vi "Autonomous Independent.vi"   [LabVIEW 2015]
doc: "This VI is called when autonomous begins, and will automatically be terminated when autonomous ends. You can carry out timed or sensor driven robot movement independently without needing to return to the caller."
uses:
  <vilib>/Rock Robotics/WPI/CAN/TalonSRX/WPI_CANTalonSRX_APIFeedbackSelect.ctl
  <vilib>/Rock Robotics/WPI/CAN/TalonSRX/WPI_CANTalonSRX_APIControlMode.ctl
  <vilib>/Rock Robotics/Network Tables/SD Read Number.vi
  <vilib>/Rock Robotics/WPI/Utilities/WPI_GetSetVariantRefNum.vi
  <vilib>/Rock Robotics/Network Tables/NT Read Number.vi
  <vilib>/Rock Robotics/WPI/RobotDrive/WPI_RobotDriveArcadeDrive_Standard(NoSaturation).vi
panel:
  # "Be sure to right-click and choose Data Operations>>Make Current Value default if you want to save the array values with the VI"
types:
  T1 = typedef "WPI_MotorControlDeviceRef.ctl" = cluster{"DeviceStatus":errorcluster, "Type":T2, "PWM":cluster{"PWM Channel":T3, "DeadBand":T4}, "CAN":cluster{"Device Number":u8, "Control Mode":T5, "Semaphore":T6, "Max Vout":dbl, "TalonSRX Control Mode":T7}, "Invert":bool}
  T2 = typedef "WPI_MotorControlType.ctl" = enum16{"PWM", "CAN", "CANTalonSRX"}
  T3 = typedef "FPGA_DIOPWMChannel.ctl" = enum8{"PWM 0", "PWM 1", "PWM 2", "PWM 3", "PWM 4", "PWM 5", "PWM 6", "PWM 7", "PWM 8", "PWM 9", "PWM MXP 0", "PWM MXP 1", "PWM MXP 2", "PWM MXP 3", "PWM MXP 4", "PWM MXP 5", "PWM MXP 6", "PWM MXP 7", "PWM MXP 8", "PWM MXP 9", "Invalid"}
  T4 = typedef "WPI_PWMDeadband.ctl" = cluster{"Name":string, "maxPositivePwm":i32, "minPositivePwm":i32, "centerPwm":i32, "maxNegativePwm":i32, "minNegativePwm":i32, "angularRange":u16}
  T5 = typedef "WPI_CANJaguar_ControlMode.ctl" = enum8{"Percent VBus", "Current", "Speed", "Position", "Voltage"}
  T6 = typedef "Semaphore RefNum" = refnum<k1>
  T7 = typedef "WPI_CANTalonSRX_APIControlMode.ctl" = enum8{"Percent VBus", "Speed", "Position", "Slave", "Unchanged / Invalid", "Voltage Compensation", "Current", "Motion Profile"}
  T8 = typedef "WPI_SwitchDevRef.ctl" = cluster{"DevStatus":errorcluster, "DIO Channel":T9, "CntIndex":T10, "Normally Closed":bool}
  T9 = typedef "FPGA_DIOChannel.ctl" = enum8{"DIO 0", "DIO 1", "DIO 2", "DIO 3", "DIO 4", "DIO 5", "DIO 6", "DIO 7", "DIO 8", "DIO 9", "DIO MXP 0", "DIO MXP 1", "DIO MXP 2", "DIO MXP 3", "DIO MXP 4", "DIO MXP 5", "DIO MXP 6", "DIO MXP 7", "DIO MXP 8", "DIO MXP 9", "DIO MXP 10", "DIO MXP 11", "DIO MXP 12", "DIO MXP 13", "DIO MXP 14", "DIO MXP 15", "Invalid"}
  T10 = typedef "FPGA_CounterCtrSystemIndex.ctl" = enum8{"Ctr 0", "Ctr 1", "Ctr 2", "Ctr 3", "Ctr 4", "Ctr 5", "Ctr 6", "Ctr 7", "Invalid"}
  T11 = typedef "WPI_GyroDevRef.ctl" = cluster{"DevStatus":errorcluster, "Analog Channel":T12, "Offset":dbl, "Gain (VoltsPerDegree/Second)":dbl, "Gyro Type":enum16{"Analog", "XRS450"}, "Handle":i32, "SPI Bus":T13, "Device Found":bool, "Sample Rate":dbl, "Calibrate On Open":bool}
  T12 = typedef "FPGA_AIChannel.ctl" = enum8{"AI 0", "AI 1", "AI 2", "AI 3", "AI MXP 0", "AI MXP 1", "AI MXP 2", "AI MXP 3", "Invalid"}
  T13 = typedef "spi_bus.ctl" = enum16{"SPI On-Board, CS0", "SPI On-Board, CS1", "SPI On-Board, CS2", "SPI On-Board, CS3", "SPI MXP", "Invalid"}
  T14 = typedef "WPI_RobotDriveDevRef.ctl" = cluster{"DevStatus":errorcluster, "Motors[]":T1[], "Square Inputs":bool, "Max Output":dbl}
  T15 = typedef "WPI_EncoderDevRef.ctl" = cluster{"DevStatus":errorcluster, "EncoderIndex":T16, "CounterIndex":T10, "DistancePerCount":dbl, "Decoding Type":T17}
  T16 = typedef "FPGA_EncoderIdx.ctl" = enum8{"Enc 0", "Enc 1", "Enc 2", "Enc 3", "Enc 4", "Enc 5", "Enc 6", "Enc 7", "Invalid"}
  T17 = typedef "WPI_EncoderType.ctl" = enum16{"1x", "2x", "4x"}
  T18 = typedef "WPI_CANTalonSRX_APIFeedbackSelect.ctl" = enum16{"Digital Quadrature Encoder", "Analog Potentiometer", "Analog Encoder", "Count on Quad-A (Rising-Edge)", "Count on Quad-A (Falling-Edge)", "CTR Magnetic Enc (Absolute)", "CTR Magnetic Enc (Relative)", "Pulse Width"}
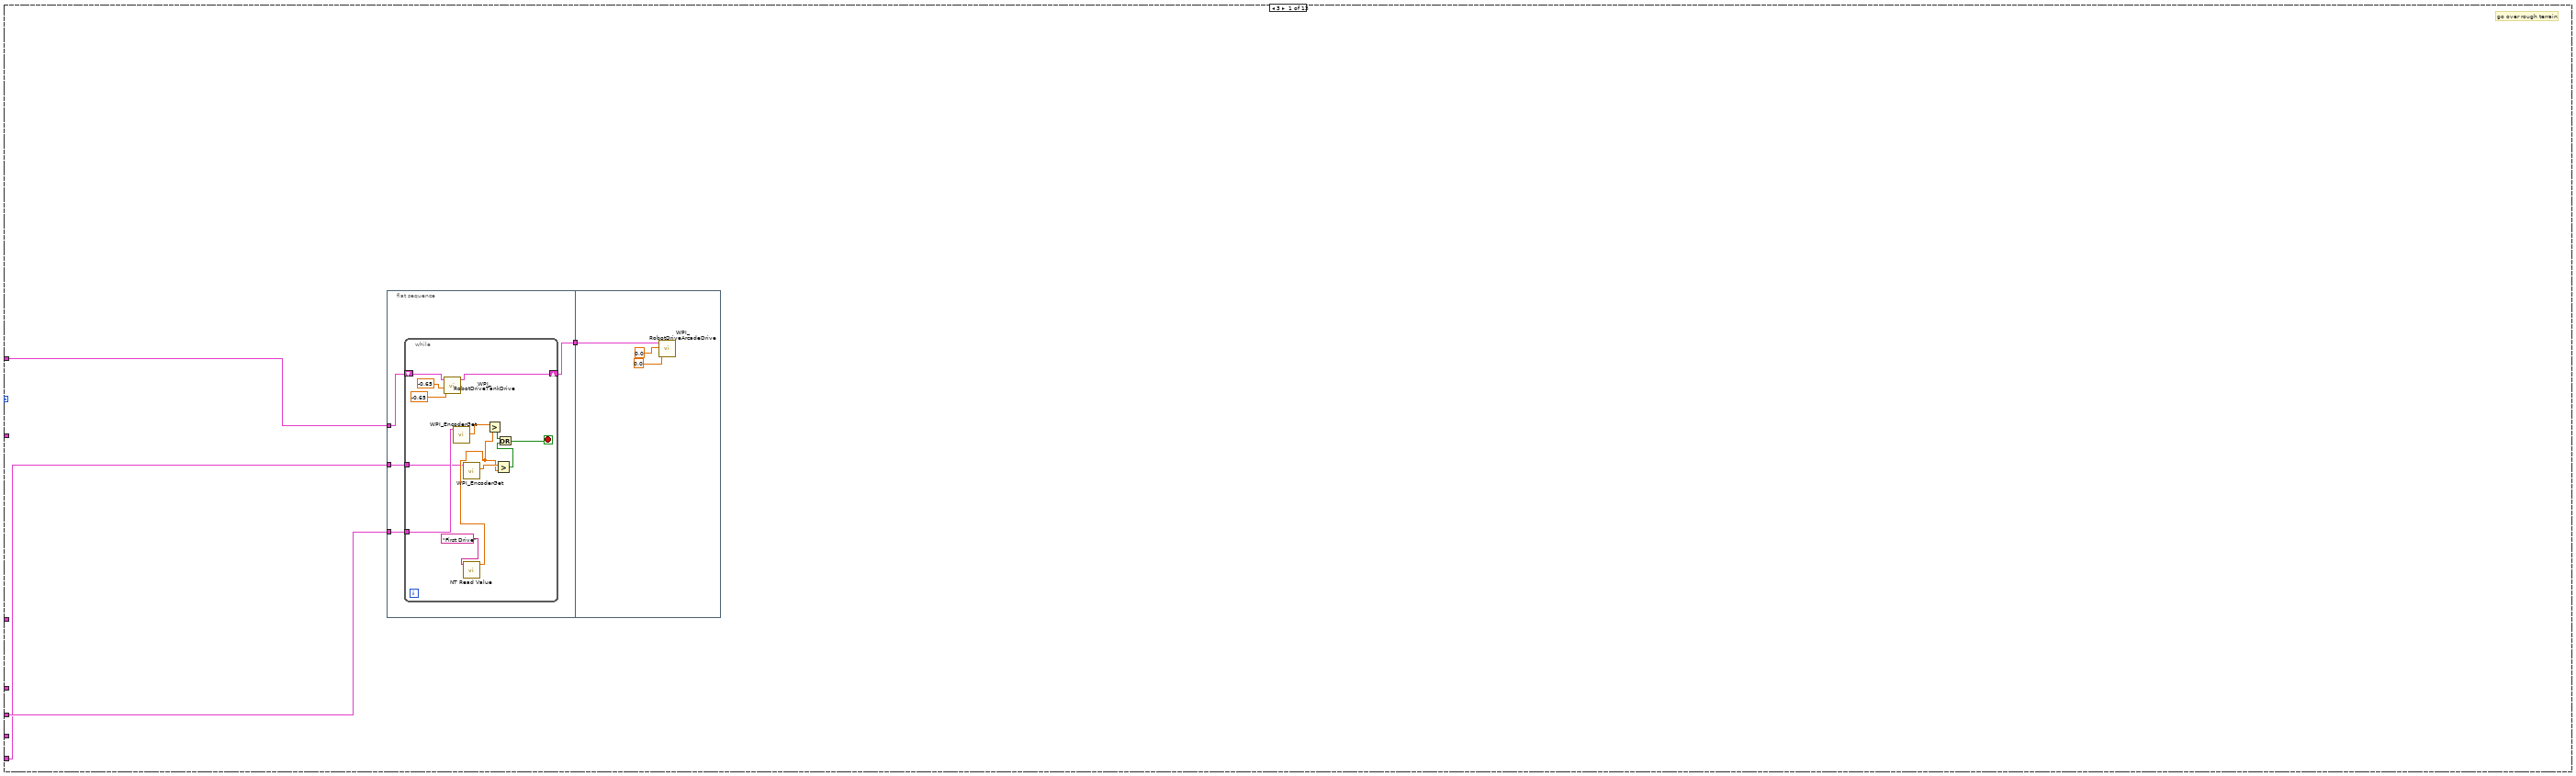
[diagram p2: hidden frame]
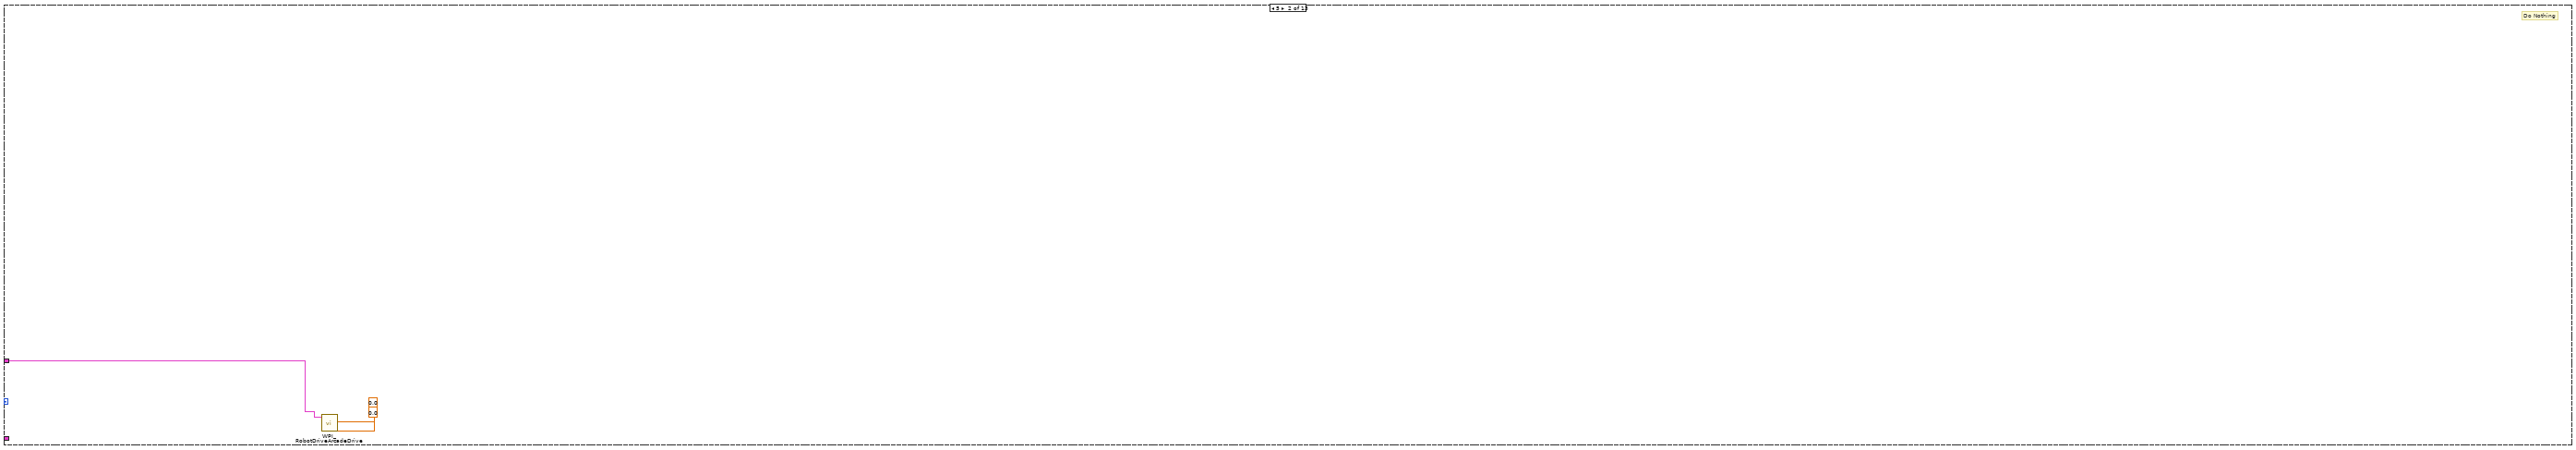
[diagram p3: hidden frame]
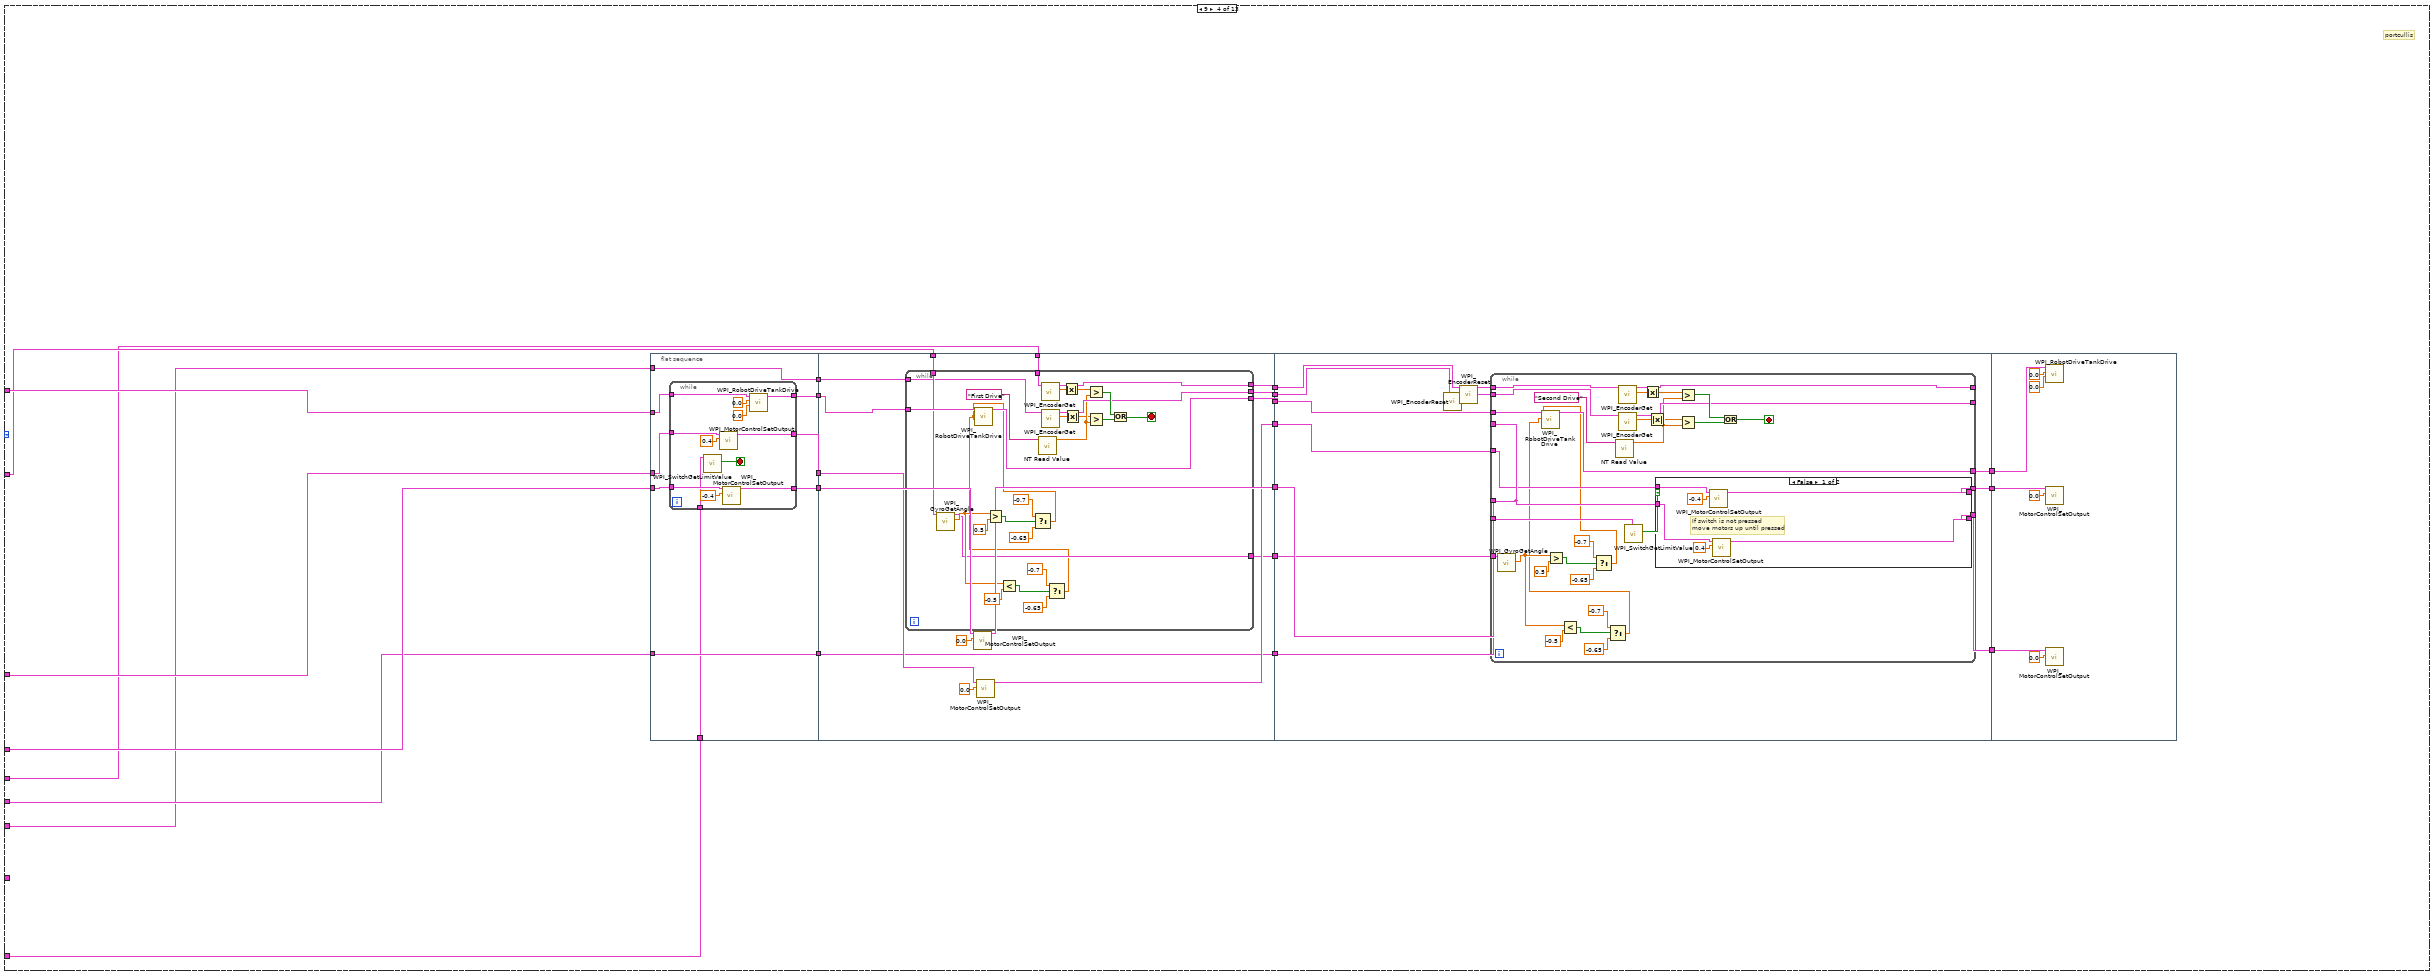
[diagram p4: hidden frame]
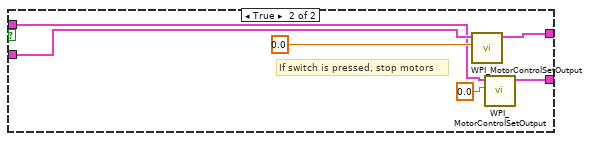
[diagram p5: hidden frame]
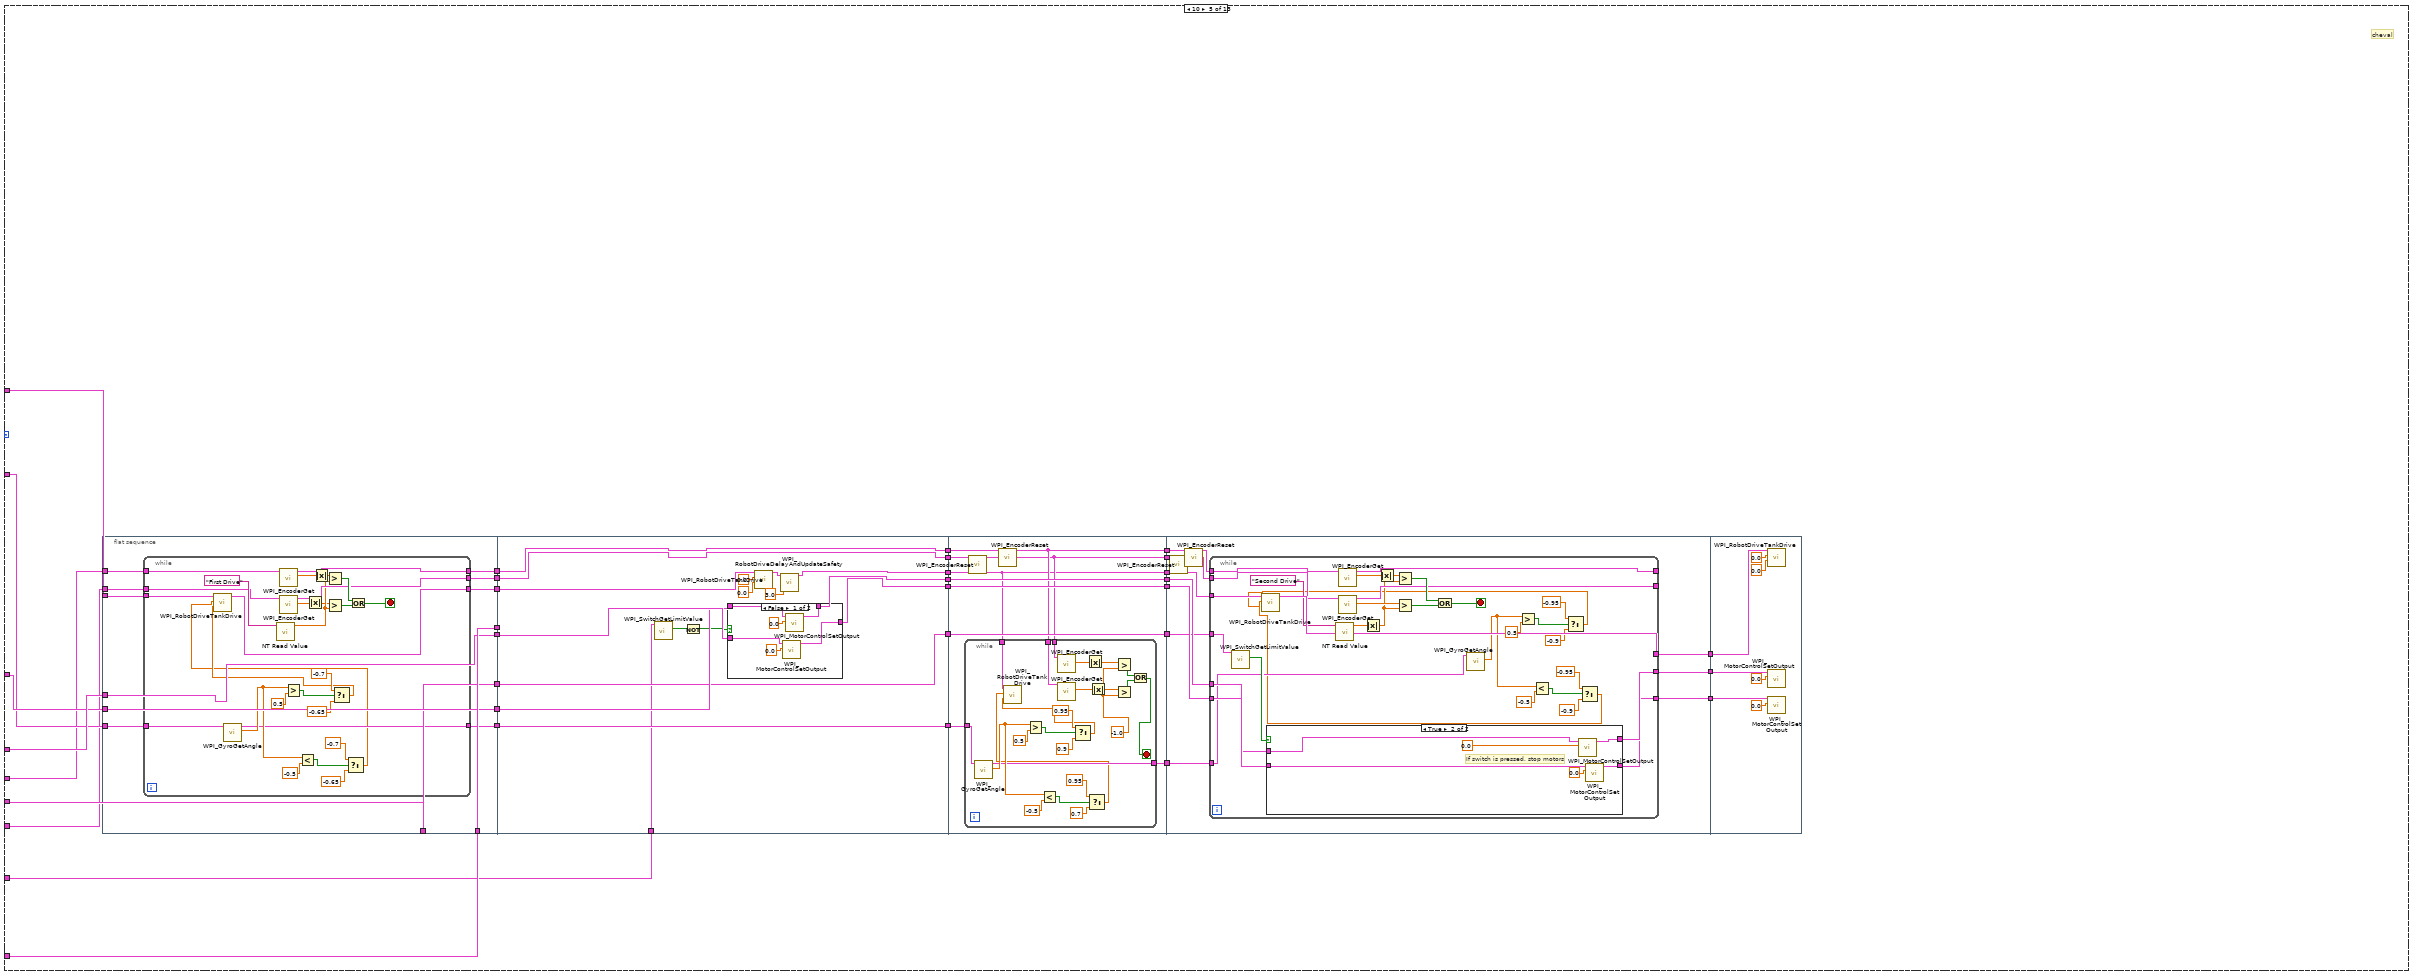
[diagram p6: hidden frame]
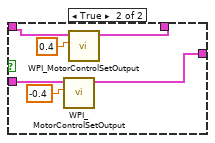
[diagram p7: hidden frame]
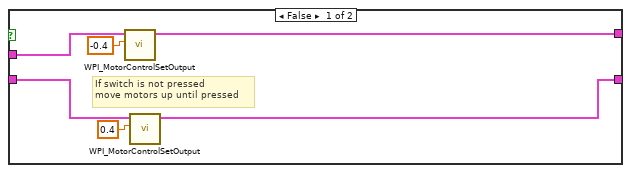
[diagram p8: hidden frame]
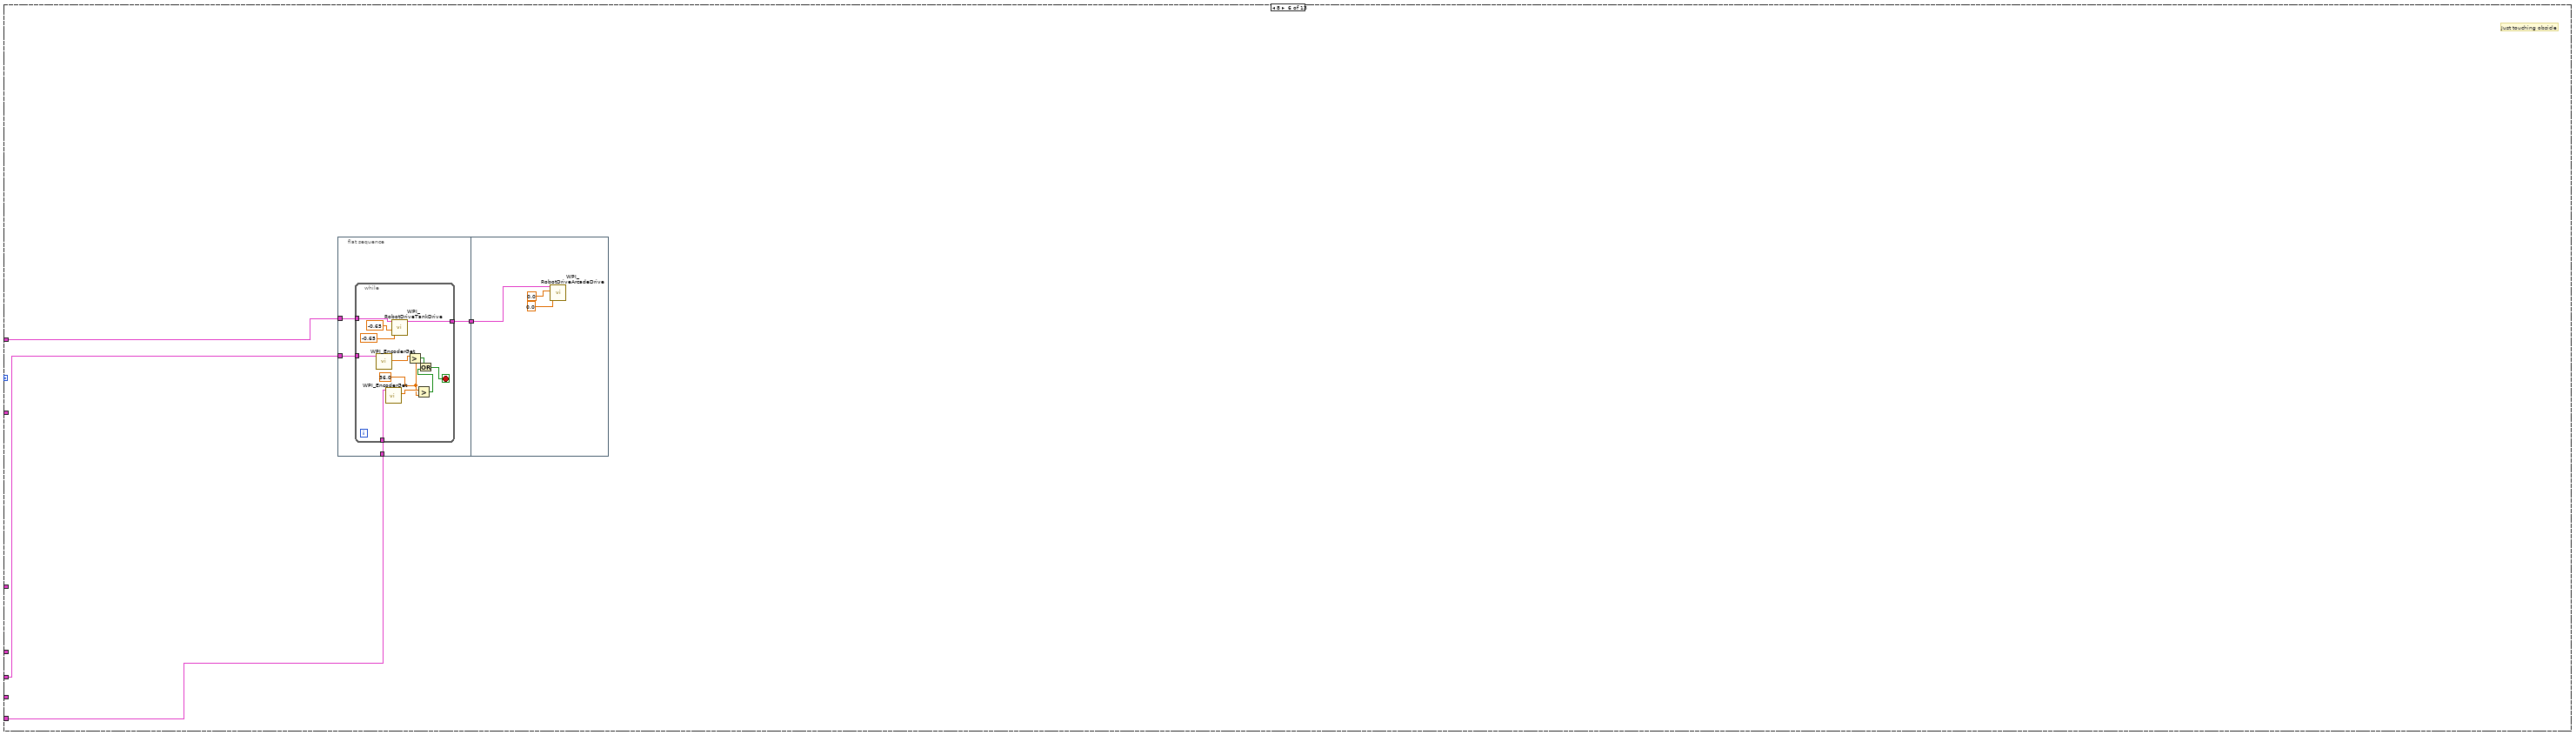
[diagram p9: hidden frame]
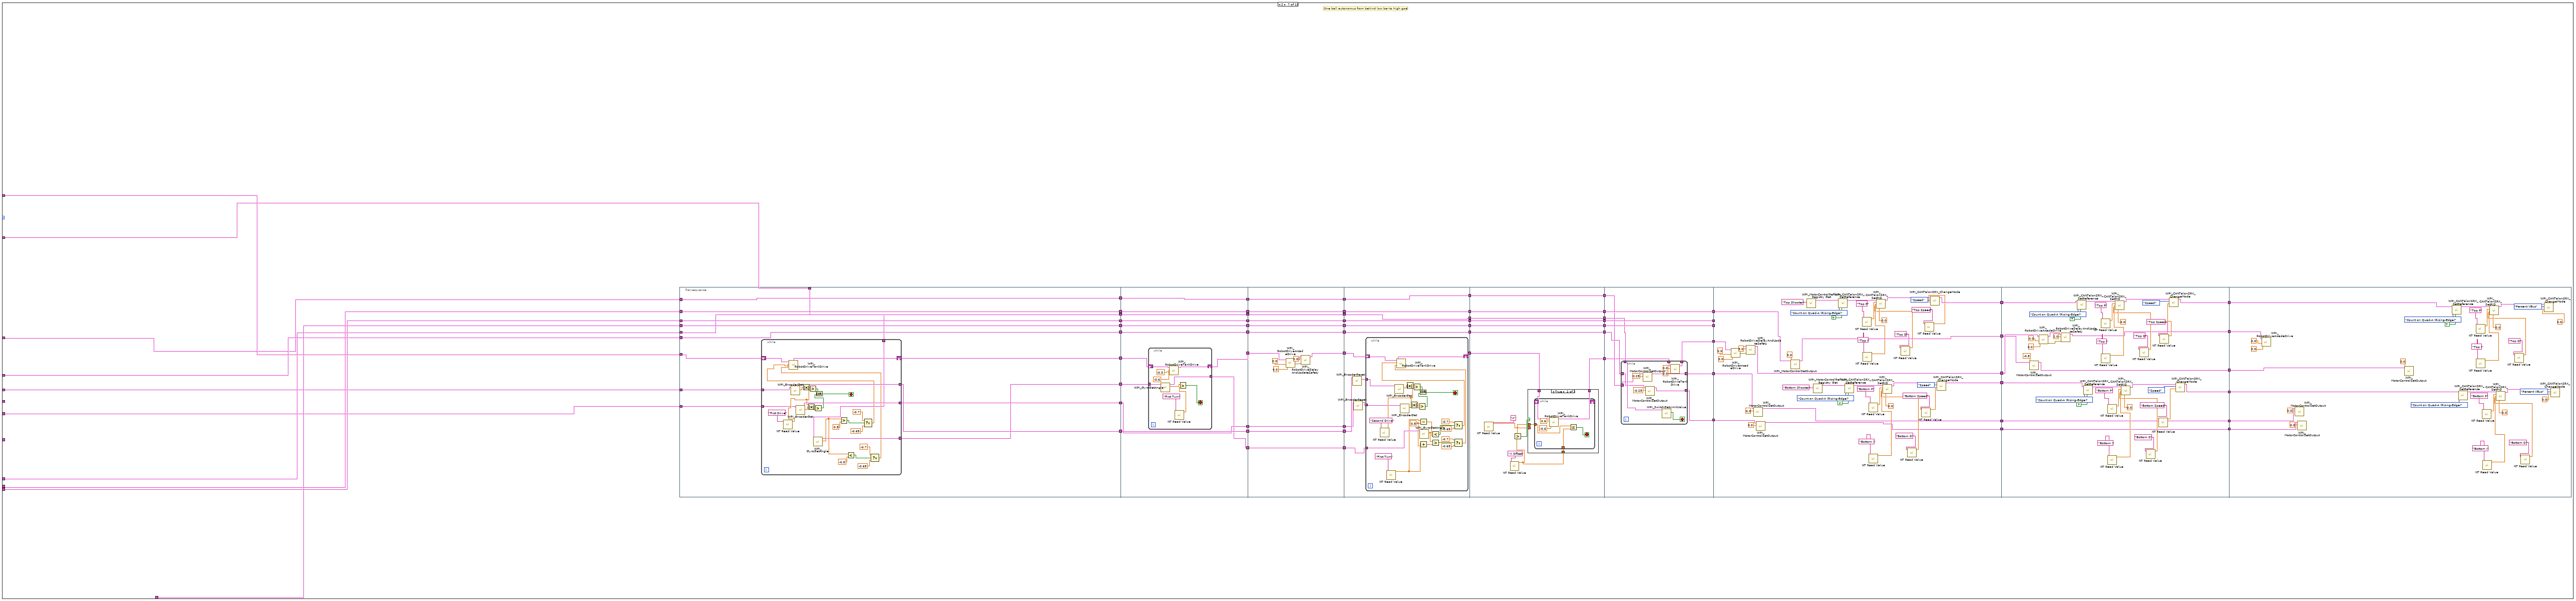
[diagram p10: hidden frame]
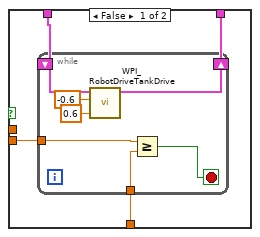
[diagram p11: hidden frame]
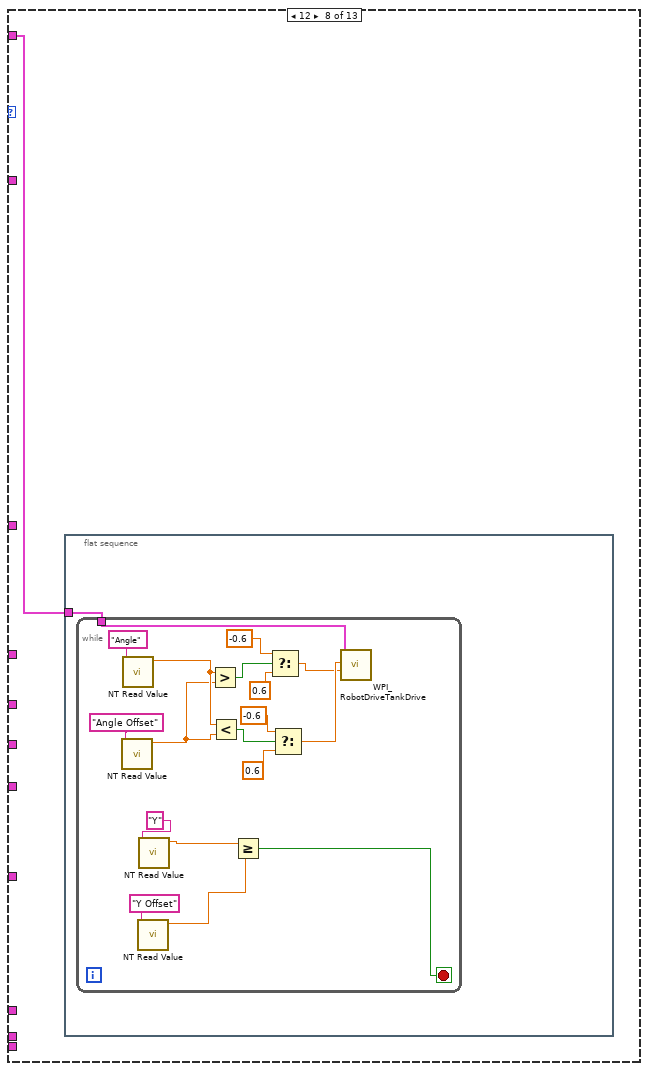
[diagram p12: hidden frame]
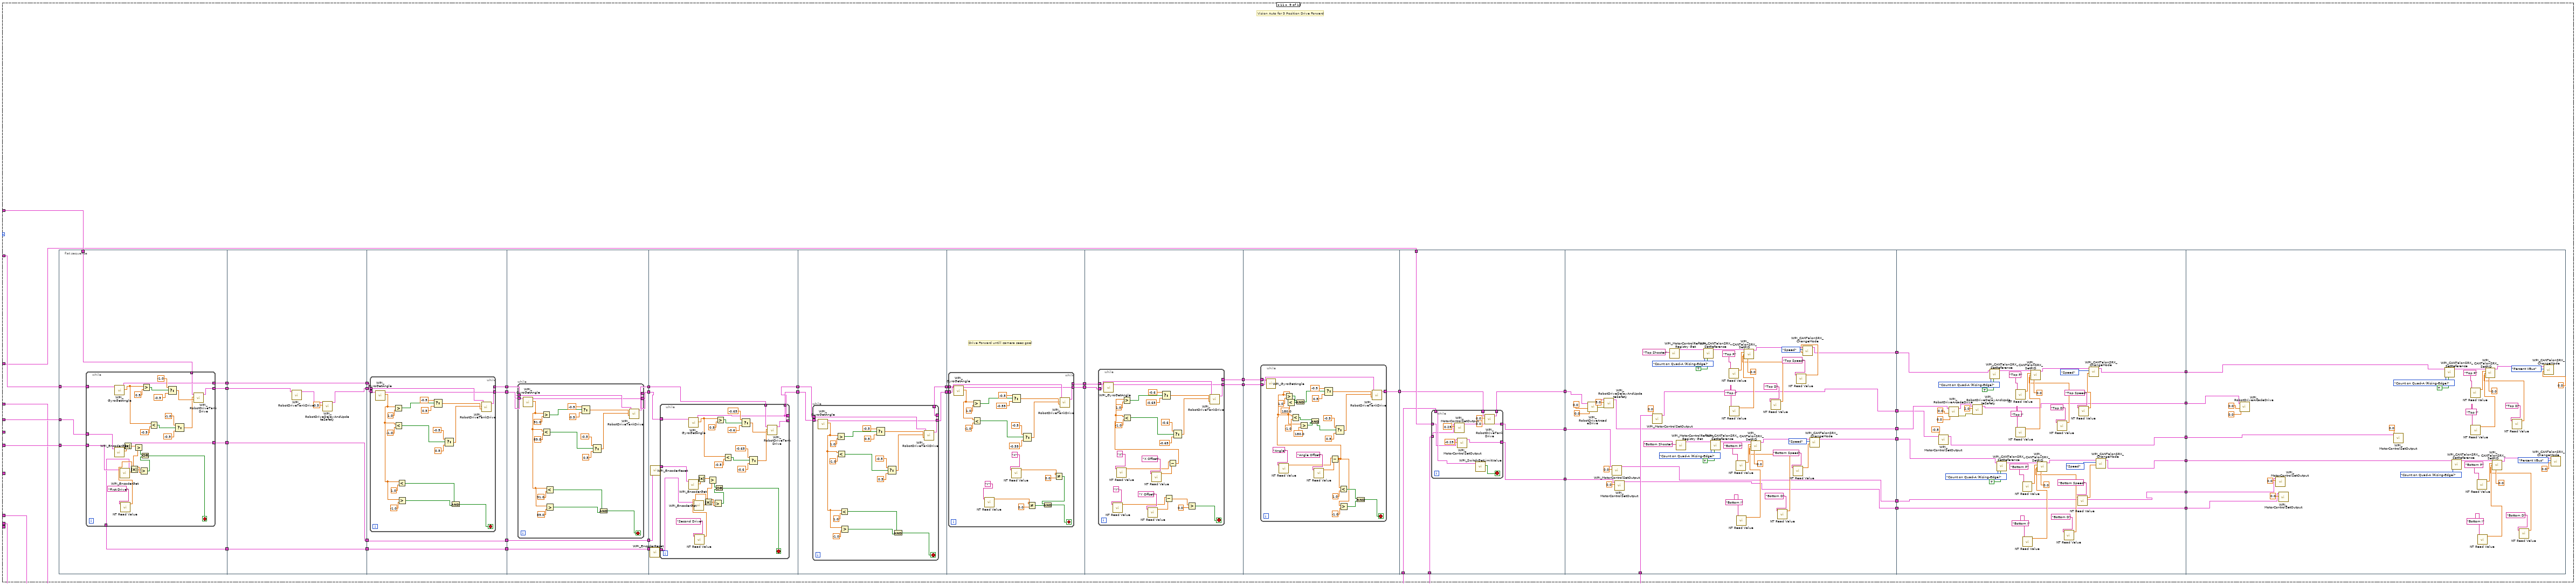
[diagram p13: hidden frame]
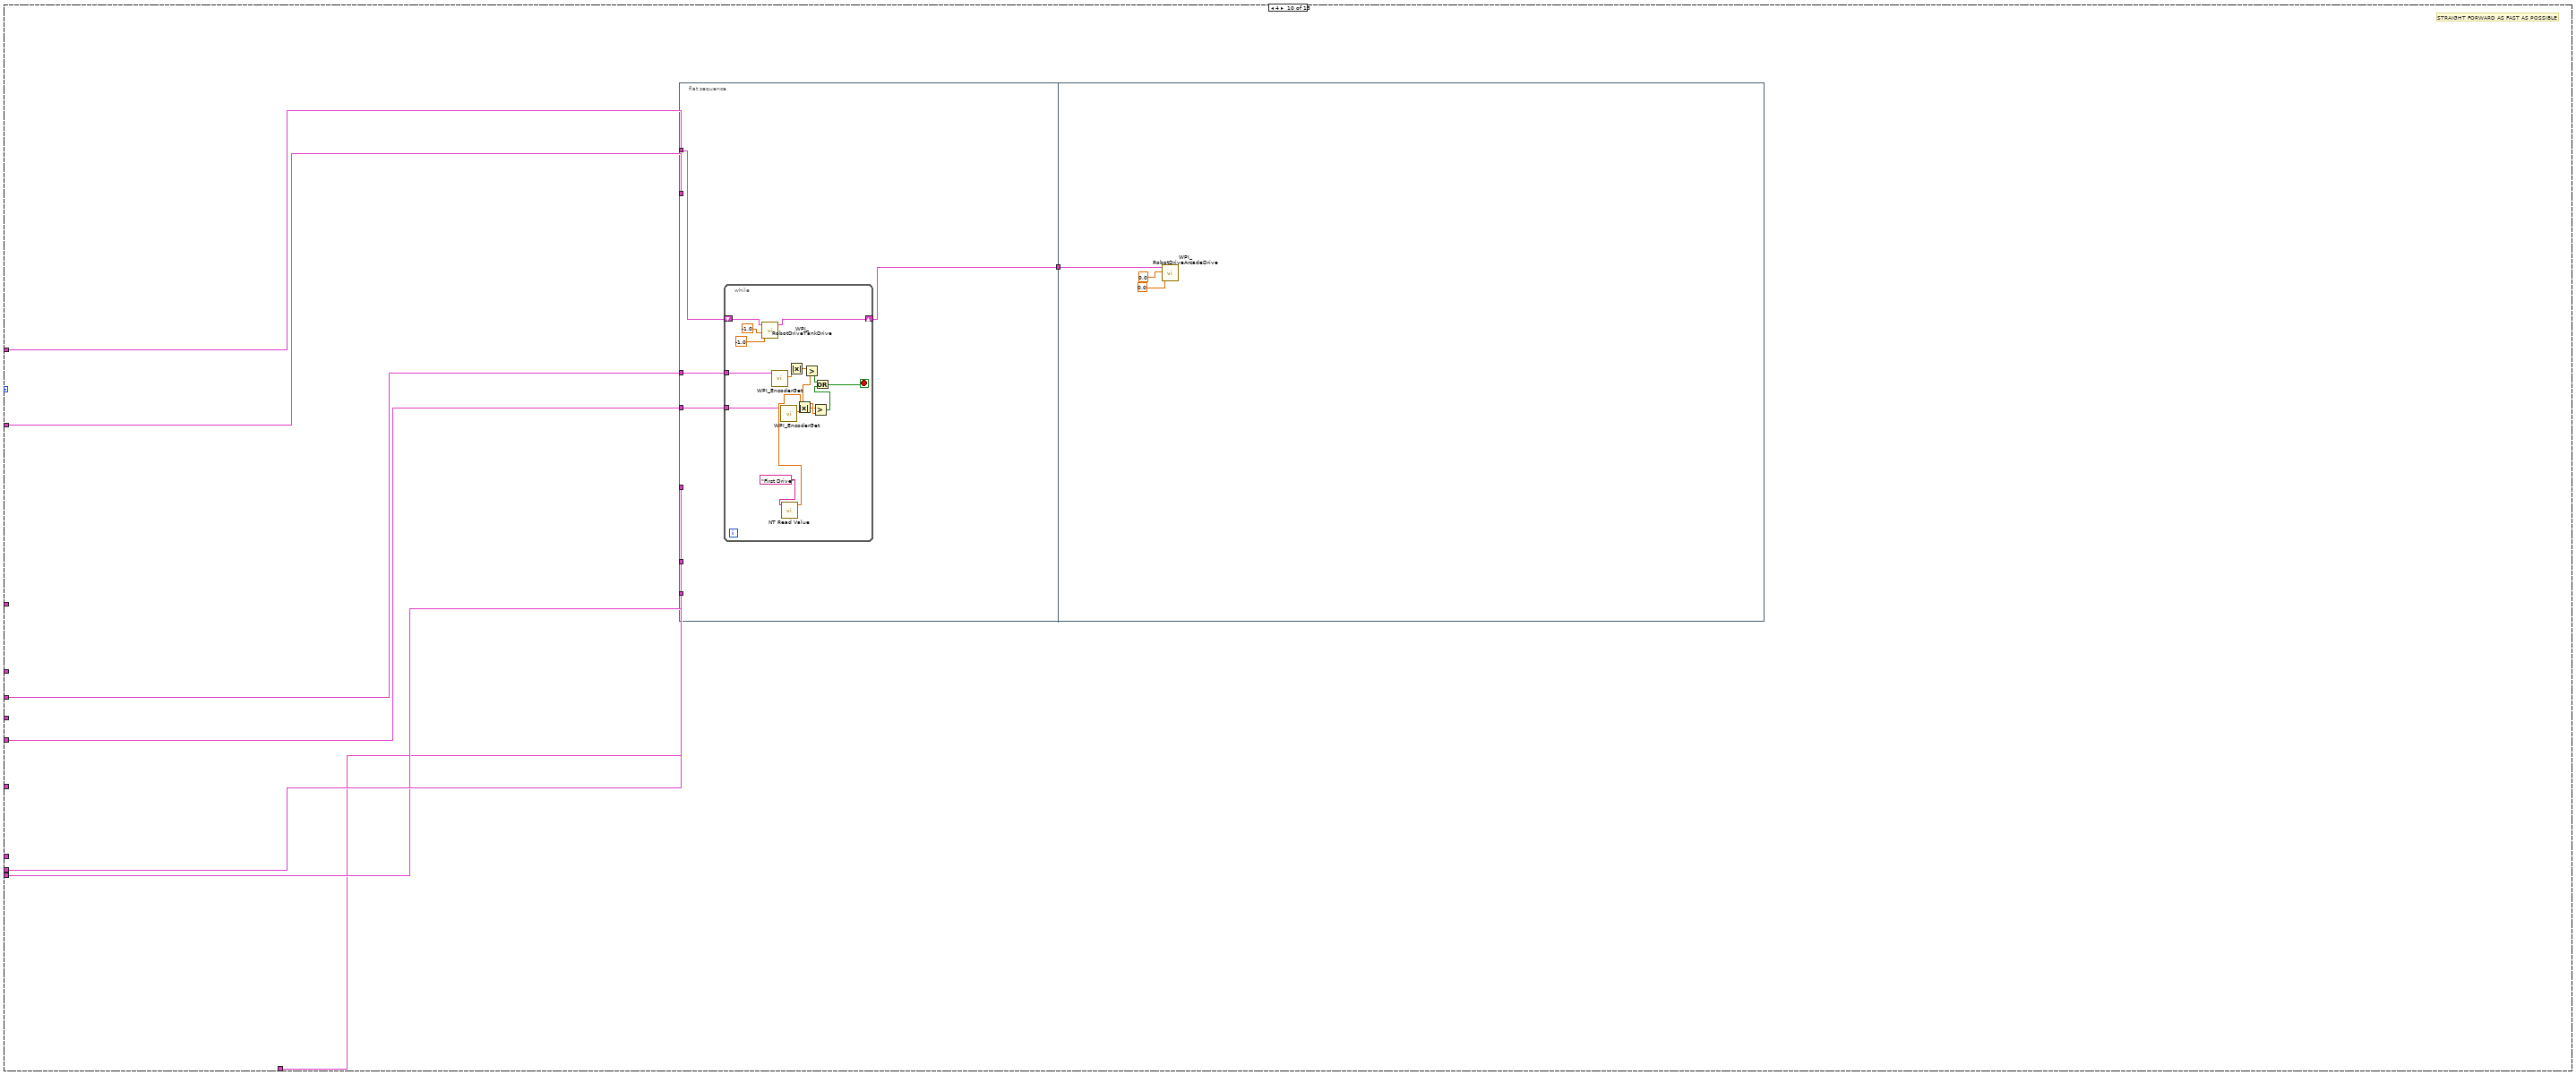
[diagram p14: hidden frame]
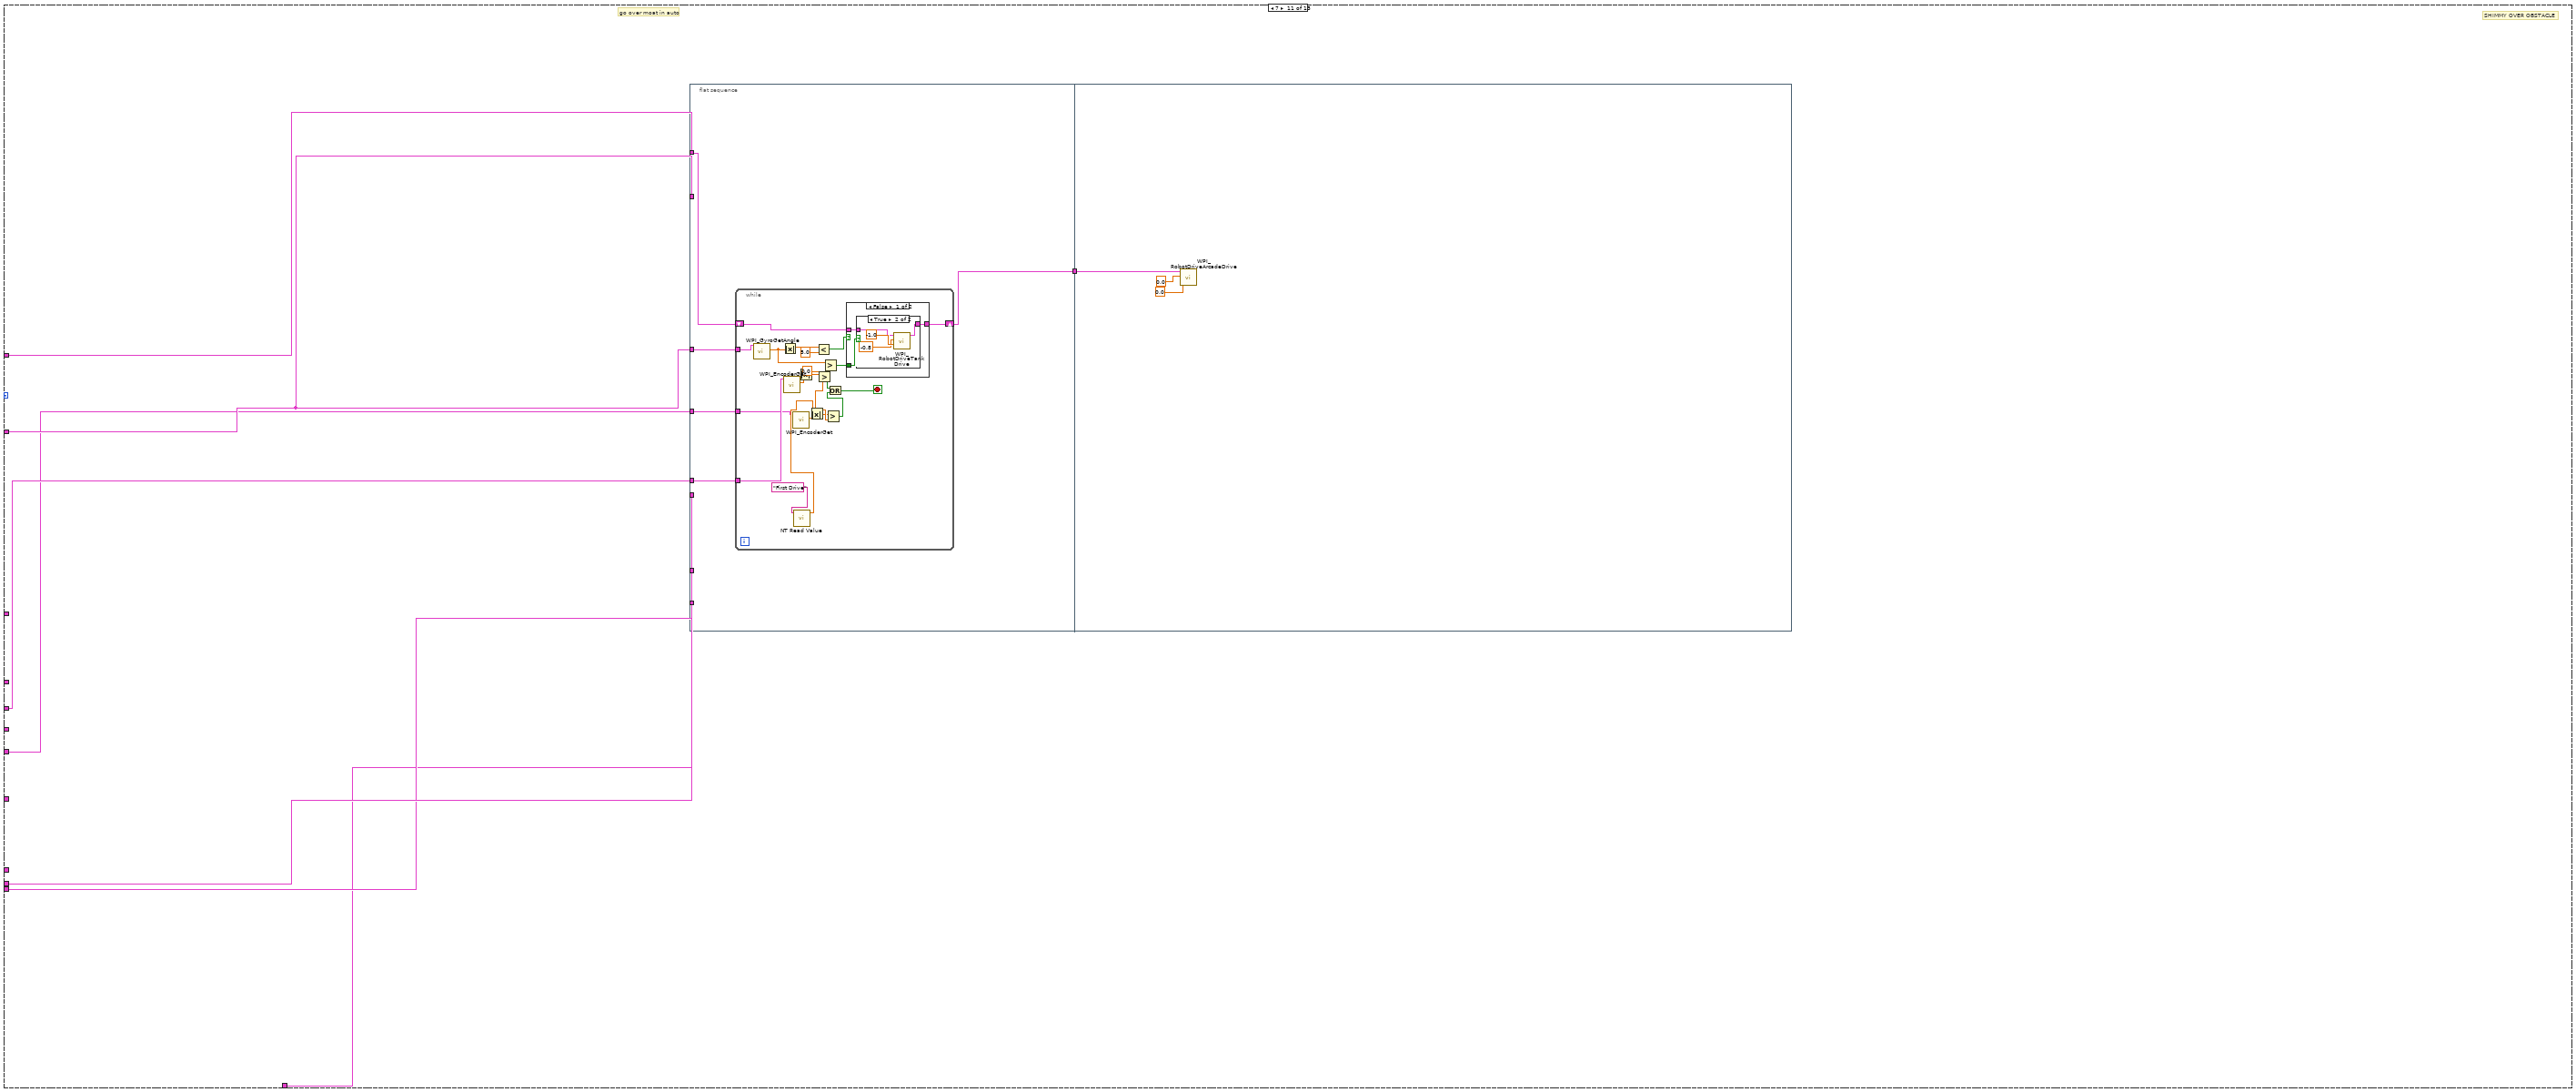
[diagram p15: hidden frame]
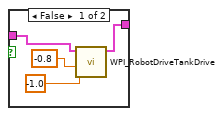
[diagram p16: hidden frame]
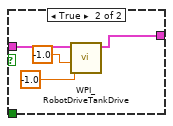
[diagram p17: hidden frame]
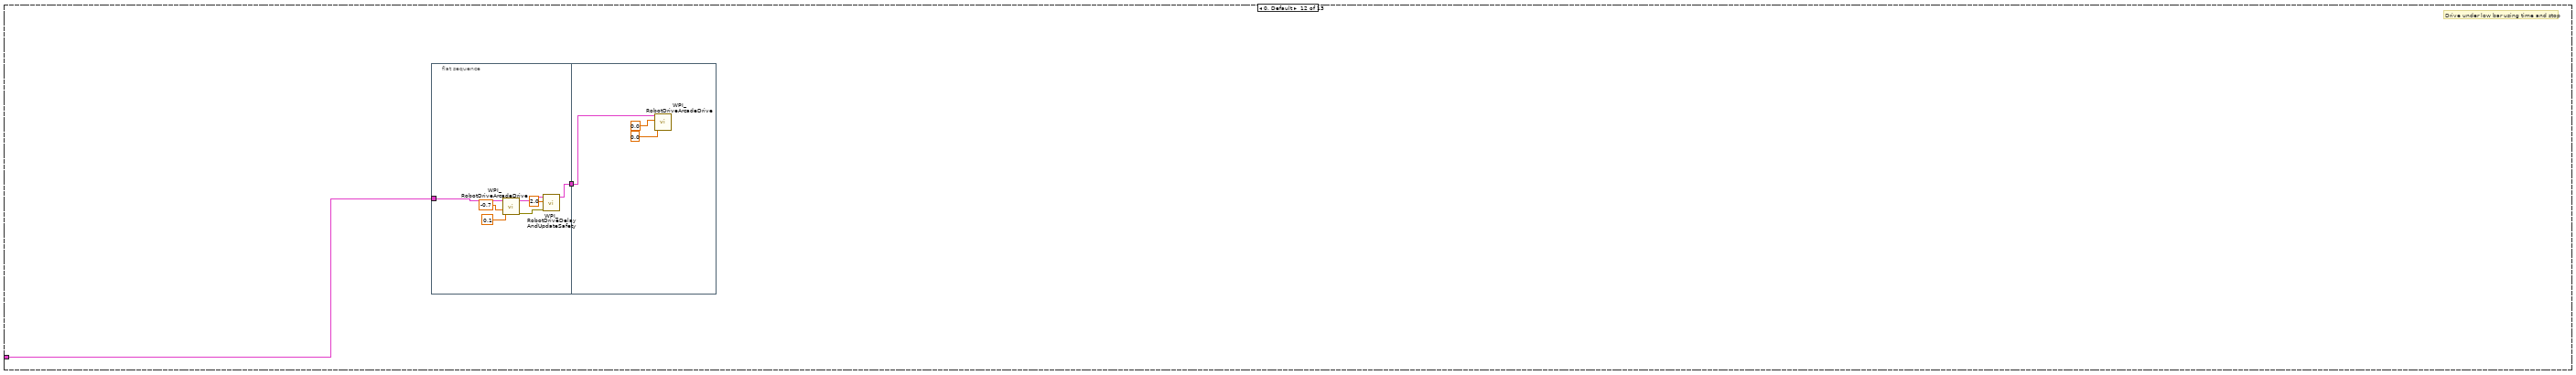
[diagram p18: hidden frame]
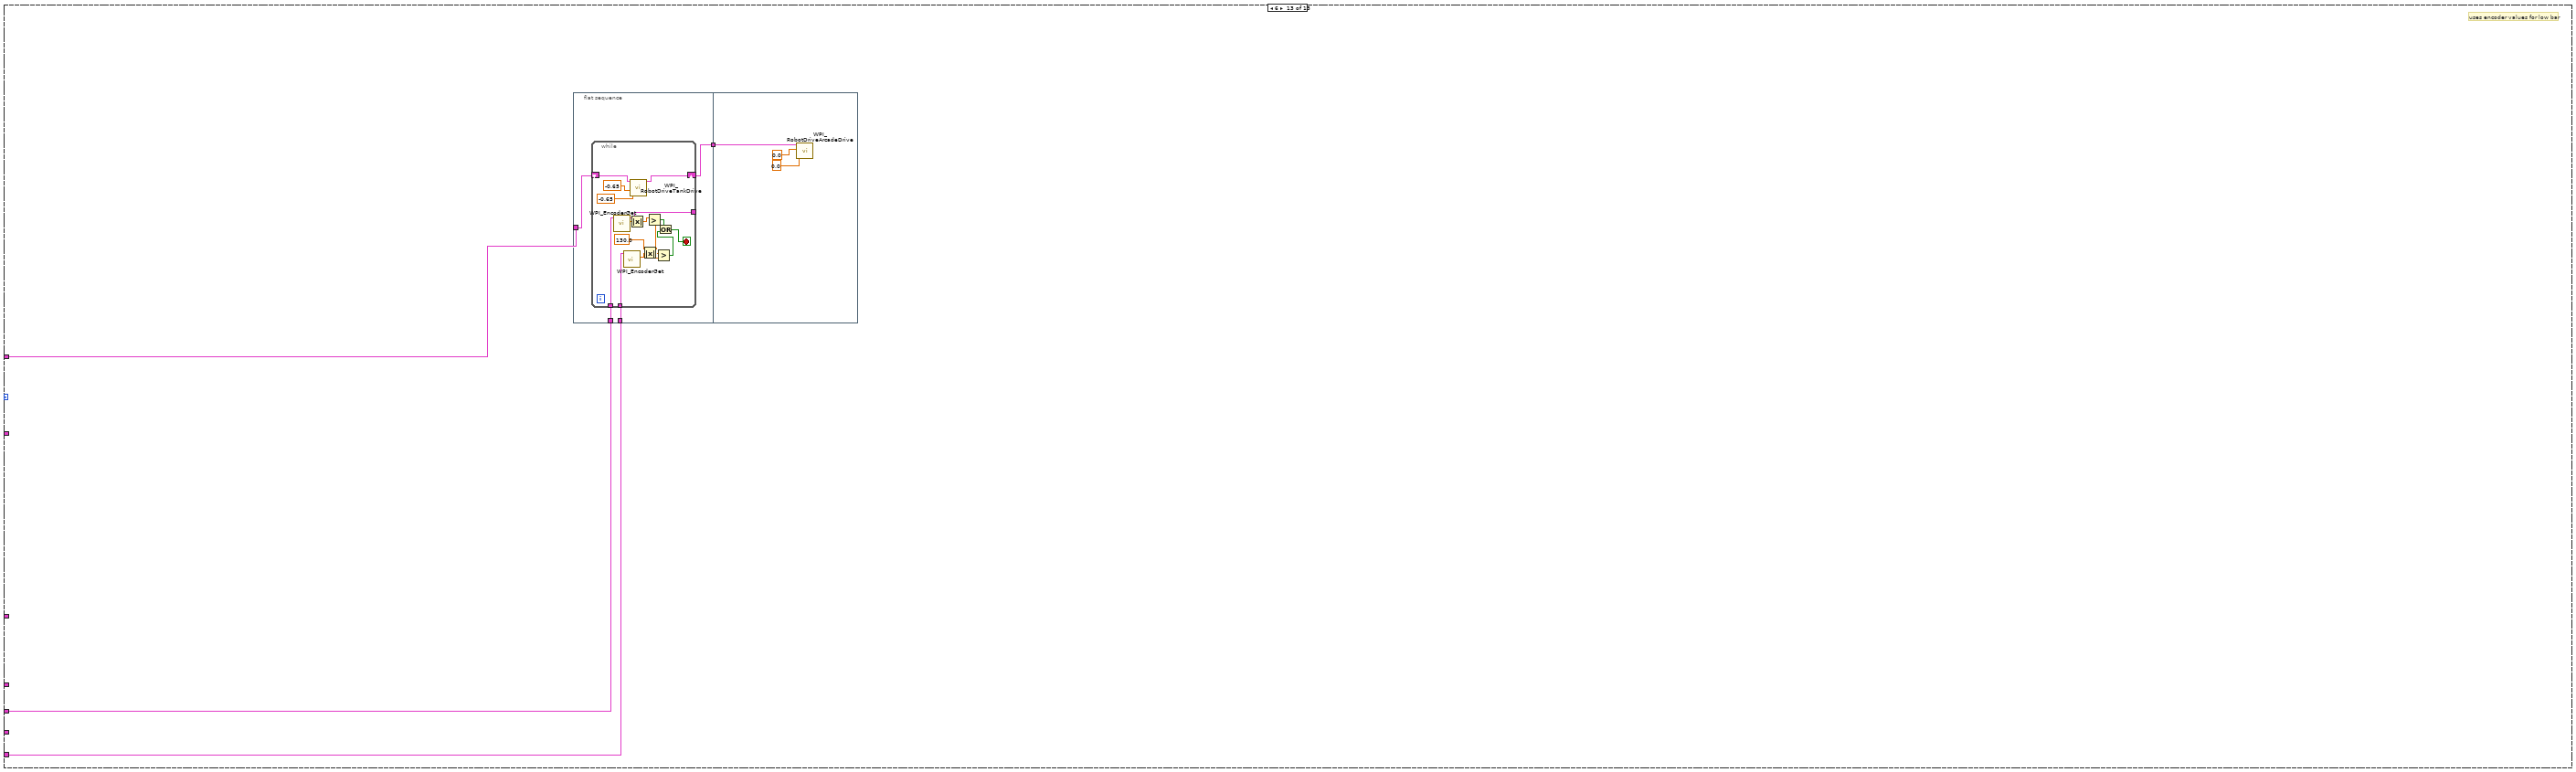
[diagram p19: hidden frame]
diagram:
  (unwired) "This function is run in parallel when the autonomous period begins. It will be terminated automatically when the period ends.\n\nNote that all Driver Station inputs are automatically latched and will not change once auto begins."
  # "Use time and/or sensors to control how the robot drives."
  # "This tells you the autonomous selected\nfrom the dashboard"
  # "Every 20ms, report that we are running autonomous\ncode. Loop will abort the same time as the VI."
  # "This tells you the driver position\nand alliance color"
  n1 = while {
    stop <- FALSE stop-if-true
    n2 = call <vilib>:"WPI_DriverStationReport Robot Code State.vi"("Autonomous"=TRUE) -> ()  [unwired: 10 in, 1 out]
    n3 = Wait (ms)(milliseconds to wait=u32 20) -> ()  [unwired: 1 out]
  }
  n4 = call <vilib>:"WPI_DriverStationGet Alliance Info.vi"() -> ()  [unwired: 12 out]
  n5 = call-poly <vilib>:"SD Read Value.vi"("Name"="Autonomous Select") -> ("Numeric"=w24:dbl)  [unwired: 8 in, 2 out]
  n6 = To Unsigned Byte Integer(number=w24) -> (unsigned 8bit integer=w22:u8)
  n7 = call <vilib>:"WPI_MotorControlRefNum Registry Get.vi"("refnum name"="Top Motor") -> ("MotorControlDevRef"=w12:T1)  [unwired: 9 in, 1 out]
  n8 = call <vilib>:"WPI_MotorControlRefNum Registry Get.vi"("refnum name"="Intake Motor") -> ("MotorControlDevRef"=w17:T1)  [unwired: 9 in, 1 out]
  n9 = call <vilib>:"WPI_MotorControlRefNum Registry Get.vi"("refnum name"="Bottom Motor") -> ("MotorControlDevRef"=w19:T1)  [unwired: 9 in, 1 out]
  n10 = call <vilib>:"WPI_SwitchRefNum Registry Get.vi"("refnum name"="Top Limit") -> ("SwitchDevRef"=w4:T8)  [unwired: 9 in, 1 out]
  n11 = call <vilib>:"WPI_SwitchRefNum Registry Get.vi"("refnum name"="Bottom Limit") -> ("SwitchDevRef"=w1:T8)  [unwired: 9 in, 1 out]
  n12 = call <vilib>:"WPI_MotorControlRefNum Registry Get.vi"("refnum name"="Window Left") -> ("MotorControlDevRef"=w7:T1)  [unwired: 9 in, 1 out]
  n13 = call <vilib>:"WPI_GyroRefNum Registry Get.vi"("refnum name"="Gyro") -> ("GyroDevRef"=w27:T11)  [unwired: 9 in, 1 out]
  n14 = call <vilib>:"WPI_MotorControlRefNum Registry Get.vi"("refnum name"="Window Right") -> ("MotorControlDevRef"=w8:T1)  [unwired: 9 in, 1 out]
  n15 = call <vilib>:"WPI_RobotDriveRefNum Registry Get.vi"("refnum name"="Drive") -> ("RobotDriveDevRef"=w28:T14)  [unwired: 9 in, 1 out]
  n16 = call <vilib>:"WPI_EncoderRefNum Registry Get.vi"("refnum name"="Right Drive Encoder") -> ("EncoderDevRef"=w26:T15)  [unwired: 9 in, 1 out]
  n17 = call <vilib>:"WPI_EncoderRefNum Registry Get.vi"("refnum name"="Left Drive Encoder") -> ("EncoderDevRef"=w25:T15)  [unwired: 9 in, 1 out]
  n18 = call <vilib>:"WPI_GyroReset.vi"("GyroDevRef"=w27) -> ("GyroDevRef"=w11:T11)  [unwired: 9 in, 1 out]
  n19 = call <vilib>:"WPI_EncoderReset.vi"("EncoderDevRef"=w25) -> ("EncoderDevRef"=w3:T15)  [unwired: 9 in, 1 out]
  n20 = call <vilib>:"WPI_EncoderReset.vi"("EncoderDevRef"=w26) -> ("EncoderDevRef"=w2:T15)  [unwired: 9 in, 1 out]
  n21 = case shown="1" w22 {
    tunnel: w28 -> [w34 w58 w101 w317 w481 w658 w749 w1058 w1118 w1522 w1552 w1599 w1614]
    tunnel: w11 -> [_ _ w61 w307 w460 _ w725 _ w1123 w1521 w1550 _ _]
    tunnel: w12 -> [_ _ w99 _ _ _ w747 _ _ w1524 w1554 _ _]
    tunnel: w19 -> [_ _ w98 _ _ _ w746 _ _ w1523 w1553 _ _]
    tunnel: w17 -> [_ _ w100 _ _ _ w748 _ w1115 w1525 w1555 _ _]
    tunnel: w8 -> [_ _ w86 w315 w476 _ w733 _ w1114 _ _ _ _]
    tunnel: w7 -> [_ _ w85 w316 w477 _ w734 _ w1113 _ _ _ _]
    tunnel: w1 -> [_ _ w84 w309 w479 _ w732 _ w1112 _ _ _ _]
    tunnel: w4 -> [_ _ _ w314 w473 _ _ _ _ _ _ _ _]
    tunnel: w3 -> [w32 _ w60 w304 w455 w655 w712 _ w1125 w1518 w1548 _ w1611]
    tunnel: w2 -> [w33 _ w59 w305 w456 w656 w713 _ w1124 w1519 w1549 _ w1612]
    tunnel: w1 -> [_ _ _ _ w454 _ _ _ _ _ _ _ _]
    frame 3 {
      # "go over rough terrain"
      n22 = flat-sequence {
        tunnel: w34 -> [w39]
        tunnel: [w38] -> w35
        tunnel: w33 -> [w37]
        tunnel: w32 -> [w36]
        tunnel: w35 -> [w53]
        frame #0 {
          n23 = while {
            shift-right: [w49] -> w38
            shift-left: w39 -> [w51]
            tunnel: w37 -> [w41]
            tunnel: w36 -> [w40]
            stop <- w42 stop-if-true
            n24 = call <vilib>:"WPI_RobotDriveTankDrive.vi"("Right axis value"=-0.65 ("Y axis value"), "Left axis value"=-0.65 ("X axis value"), "RobotDriveDevRef"=w51) -> ("RobotDriveDevRef"=w49:T14)  [unwired: 6 in, 2 out]
            n25 = call <vilib>:"WPI_EncoderGet.vi"("EncoderDevRef"=w41) -> ("Distance"=w45:dbl)  [unwired: 5 in, 5 out]
            n26 = call <vilib>:"WPI_EncoderGet.vi"("EncoderDevRef"=w40) -> ("Distance"=w47:dbl)  [unwired: 5 in, 5 out]
            n27 = call-poly <vilib>:"NT Read Value.vi"("Name"="First Drive") -> ("Numeric"=w44:dbl)  [unwired: 9 in, 1 out]
            n28 = Greater?(x=w45, y=w44) -> (0:w43:bool)
            n29 = Greater?(x=w47, y=w44) -> (0:w46:bool)
            n30 = Or(x=w43, y=w46) -> (x .or. y?=w42:bool)
          }
        }
        frame #1 {
          n31 = call-poly <vilib>:"WPI_RobotDriveArcadeDrive.vi"("Y axis value"=0.0, "X axis value"=0.0, "RobotDriveDevRef"=w53) -> ()  [unwired: 6 in, 3 out]
        }
      }
    }
    frame 5 {
      # "Do Nothing"
      n32 = call-poly <vilib>:"WPI_RobotDriveArcadeDrive.vi"("Y axis value"=0.0, "X axis value"=0.0, "RobotDriveDevRef"=w58) -> ()  [unwired: 6 in, 3 out]
    }
    frame 1 {
      # "One ball autonomus from behind low bar to low goal"
      n33 = flat-sequence {
        tunnel: [w113] -> w77
        tunnel: [w112] -> w75
        tunnel: [w111] -> w73
        tunnel: [w110] -> w71
        tunnel: [w109] -> w69
        tunnel: [w108] -> w67
        tunnel: [w106] -> w65
        tunnel: [w107] -> w64
        tunnel: w61 -> [w107]
        tunnel: w84 -> [w108]
        tunnel: w85 -> [w109]
        tunnel: w86 -> [w110]
        tunnel: w98 -> [w111]
        tunnel: w99 -> [w112]
        tunnel: w100 -> [w113]
        tunnel: w101 -> [w105]
        tunnel: w61 -> [w104]
        tunnel: w60 -> [w103]
        tunnel: w59 -> [w102]
        tunnel: w77 -> [w149]
        tunnel: [w149] -> w76
        tunnel: w75 -> [w148]
        tunnel: [w148] -> w74
        tunnel: w73 -> [w147]
        tunnel: [w147] -> w72
        tunnel: w71 -> [w146]
        tunnel: [w146] -> w70
        tunnel: w69 -> [w145]
        tunnel: [w145] -> w68
        tunnel: w67 -> [w144]
        tunnel: [w144] -> w66
        tunnel: w65 -> [w143]
        tunnel: w64 -> [w142]
        tunnel: [w141] -> w62
        tunnel: w76 -> [w170]
        tunnel: [w170] -> w89
        tunnel: w74 -> [w169]
        tunnel: [w169] -> w88
        tunnel: w72 -> [w168]
        tunnel: [w168] -> w87
        tunnel: w70 -> [w167]
        tunnel: w68 -> [w166]
        tunnel: w66 -> [w165]
        tunnel: [w164] -> w83
        tunnel: [w163] -> w82
        tunnel: [w159] -> w63
        tunnel: w62 -> [w160]
        tunnel: [w225] -> w97
        tunnel: w89 -> [w187]
        tunnel: w88 -> [_]
        tunnel: w87 -> [_]
        tunnel: [w190] -> w96
        tunnel: [w189] -> w94
        tunnel: [w186] -> w91
        tunnel: w83 -> [w183]
        tunnel: w82 -> [w182]
        tunnel: [w181] -> w81
        tunnel: [w180] -> w78
        tunnel: w63 -> [w179]
        tunnel: w97 -> [w241]
        tunnel: w96 -> [w236]
        tunnel: [w235] -> w95
        tunnel: w94 -> [w238]
        tunnel: [w240] -> w93
        tunnel: [w239] -> w92
        tunnel: w91 -> [w230]
        tunnel: [w228] -> w90
        tunnel: w81 -> [w227]
        tunnel: [w227] -> w80
        tunnel: [w226] -> w79
        tunnel: w78 -> [w226]
        tunnel: w95 -> [w277]
        tunnel: w93 -> [w275]
        tunnel: w92 -> [w274]
        tunnel: w90 -> [w271]
        tunnel: w80 -> [w268]
        tunnel: w79 -> [w267]
        frame #0 {
          n34 = while {
            shift-right: [w139] -> w106
            shift-left: w105 -> [w140]
            tunnel: [w133] -> _
            tunnel: [w132] -> _
            tunnel: w104 -> [w127]
            tunnel: w103 -> [w115]
            tunnel: w102 -> [w114]
            stop <- w134 stop-if-true
            n35 = call <vilib>:"WPI_GyroGetAngle.vi"("GyroDevRef"=w127) -> ("Angle"=w119:dbl)  [unwired: 6 in, 4 out]
            n36 = call-poly <vilib>:"NT Read Value.vi"("Name"="First Drive") -> ("Numeric"=w128:dbl)  [unwired: 9 in, 1 out]
            n37 = call <vilib>:"WPI_EncoderGet.vi"("EncoderDevRef"=w114) -> ("Distance"=w136:dbl, "EncoderDevRef"=w133:T15)  [unwired: 5 in, 4 out]
            n38 = call <vilib>:"WPI_EncoderGet.vi"("EncoderDevRef"=w115) -> ("Distance"=w138:dbl, "EncoderDevRef"=w132:T15)  [unwired: 5 in, 4 out]
            n39 = Absolute Value(x=w136) -> (abs(x)=w131:dbl)
            n40 = Absolute Value(x=w138) -> (abs(x)=w130:dbl)
            n41 = Greater?(x=w119, y=0.5) -> (0:w125:bool)
            n42 = Greater?(x=w131, y=w128) -> (0:w135:bool)
            n43 = Greater?(x=w130, y=w128) -> (0:w137:bool)
            n44 = Less?(x=w119, y=-0.5) -> (x < y?=w121:bool)
            n45 = Or(x=w135, y=w137) -> (x .or. y?=w134:bool)
            n46 = Select(t=-0.7, s=w125, f=-0.65) -> (s? t:f=w117:dbl)
            n47 = Select(t=-0.7, s=w121, f=-0.65) -> (s? t:f=w116:dbl)
            n48 = call <vilib>:"WPI_RobotDriveTankDrive.vi"("Right axis value"=w117, "Left axis value"=w116, "RobotDriveDevRef"=w140) -> ("RobotDriveDevRef"=w139:T14)  [unwired: 6 in, 2 out]
          }
        }
        frame #1 {
          n49 = while {
            shift-right: [w155] -> w141
            shift-left: w143 -> [w157]
            tunnel: w142 -> [w152]
            stop <- w153 stop-if-true
            n50 = call <vilib>:"WPI_GyroGetAngle.vi"("GyroDevRef"=w152) -> ("Angle"=w154:dbl)  [unwired: 6 in, 4 out]
            n51 = call-poly <vilib>:"NT Read Value.vi"("Name"="First Turn") -> ("Numeric"=w150:dbl)  [unwired: 9 in, 1 out]
            n52 = call <vilib>:"WPI_RobotDriveTankDrive.vi"("Right axis value"=-0.3 ("Y axis value"), "Left axis value"=-0.6 ("X axis value"), "RobotDriveDevRef"=w157) -> ("RobotDriveDevRef"=w155:T14)  [unwired: 6 in, 2 out]
            n53 = Greater Or Equal?(x=w154, y=w150) -> (x >= y?=w153:bool)
          }
        }
        frame #2 {
          n54 = while {
            tunnel: w167 -> [w178]
            tunnel: w166 -> [w177]
            tunnel: w165 -> [w174]
            tunnel: [w172] -> w164
            tunnel: [w171] -> w163
            stop <- w173 stop-if-true
            n55 = call <vilib>:"WPI_MotorControlSetOutput.vi"("Output"=0.4, "MotorControlDevRef"=w178) -> ("MotorControlDevRef"=w172:T1)  [unwired: 7 in, 2 out]
            n56 = call <vilib>:"WPI_MotorControlSetOutput.vi"("Output"=-0.4, "MotorControlDevRef"=w177) -> ("MotorControlDevRef"=w171:T1)  [unwired: 7 in, 2 out]
            n57 = call <vilib>:"WPI_SwitchGetLimitValue.vi"("SwitchDevRef"=w174) -> ("Switch Pressed"=w173:bool)  [unwired: 8 in, 2 out]
          }
          n58 = call-poly <vilib>:"WPI_RobotDriveArcadeDrive.vi"("Y axis value"=0.0, "X axis value"=0.0, "RobotDriveDevRef"=w160) -> ("RobotDriveDevRef"=w159:T14)  [unwired: 6 in, 2 out]
        }
        frame #3 {
          n59 = call-poly <vilib>:"WPI_RobotDriveArcadeDrive.vi"("Y axis value"=0.0, "X axis value"=0.0, "RobotDriveDevRef"=w179) -> ("error out"=w223:errorcluster, "RobotDriveDevRef"=w222:T14)  [unwired: 6 in, 1 out]
          n60 = call <vilib>:"WPI_MotorControlSetOutput.vi"("Output"=0.0, "MotorControlDevRef"=w183) -> ("MotorControlDevRef"=w181:T1)  [unwired: 7 in, 2 out]
          n61 = call <vilib>:"WPI_MotorControlSetOutput.vi"("Output"=0.0, "MotorControlDevRef"=w182) -> ("MotorControlDevRef"=w180:T1)  [unwired: 7 in, 2 out]
          n62 = call <vilib>:"WPI_RobotDriveDelayAndUpdateSafety.vi"("error in (no error)"=w223, "Delay (s)"=3.0, "RobotDriveDevRef"=w222) -> ("RobotDriveDevRef 2"=w186:T14)  [unwired: 7 in, 1 out]
          n63 = call <vilib>:"WPI_MotorControlSetOutput.vi"("Output"=0.0, "MotorControlDevRef"=w187) -> ("MotorControlDevRef"=w225:T1)  [unwired: 7 in, 2 out]
          n64 = call <vilib>:"WPI_MotorControlRefNum Registry Get.vi"("refnum name"="Top Shooter") -> ("MotorControlDevRef"=w217:T1)  [unwired: 9 in, 1 out]
          n65 = call <vilib>:"WPI_MotorControlRefNum Registry Get.vi"("refnum name"="Bottom Shooter") -> ("MotorControlDevRef"=w203:T1)  [unwired: 9 in, 1 out]
          n66 = call <vilib>:"WPI_CANTalonSRX_SetReference.vi"("Reverse Closed-Loop Output"=TRUE, "Feedback Reference"=WPI_CANTalonSRX_APIFeedbackSelect."Count on Quad-A (Rising-Edge)", "CAN Talon SRX Ref"=w217) -> ("CAN Talon SRX Ref"=w218:T1)  [unwired: 7 in, 1 out]
          n67 = call <vilib>:"WPI_CANTalonSRX_SetReference.vi"("Feedback Reference"=WPI_CANTalonSRX_APIFeedbackSelect."Count on Quad-A (Rising-Edge)", "CAN Talon SRX Ref"=w203) -> ("CAN Talon SRX Ref"=w204:T1)  [unwired: 8 in, 1 out]
          n68 = call-poly <vilib>:"NT Read Value.vi"("Name"="Top P") -> ("Numeric"=w209:dbl)  [unwired: 9 in, 1 out]
          n69 = call-poly <vilib>:"NT Read Value.vi"("Name"="Top I") -> ("Numeric"=w208:dbl)  [unwired: 9 in, 1 out]
          n70 = call-poly <vilib>:"NT Read Value.vi"("Name"="Bottom P") -> ("Numeric"=w195:dbl)  [unwired: 9 in, 1 out]
          n71 = call-poly <vilib>:"NT Read Value.vi"("Name"="Bottom I") -> ("Numeric"=w194:dbl)  [unwired: 9 in, 1 out]
          n72 = call-poly <vilib>:"NT Read Value.vi"("Name"="Top D") -> ("Numeric"=w207:dbl)  [unwired: 9 in, 1 out]
          n73 = call <vilib>:"WPI_CANTalonSRX_SetPID.vi"("CAN Talon SRX Ref"=w218, "P"=w209, "I"=w208, "D"=w207, "F"=0.0) -> ("CAN Talon SRX Ref"=w214:T1)  [unwired: 9 in, 1 out]
          n74 = call-poly <vilib>:"NT Read Value.vi"("Name"="Bottom D") -> ("Numeric"=w193:dbl)  [unwired: 9 in, 1 out]
          n75 = call <vilib>:"WPI_CANTalonSRX_SetPID.vi"("CAN Talon SRX Ref"=w204, "P"=w195, "I"=w194, "D"=w193, "F"=0.0) -> ("CAN Talon SRX Ref"=w200:T1)  [unwired: 9 in, 1 out]
          n76 = call <vilib>:"WPI_CANTalonSRX_ChangeMode.vi"("Output"=-0.7, "Control Mode"=WPI_CANTalonSRX_APIControlMode."Percent VBus", "CAN Talon SRX Ref"=w214) -> ("CAN Talon SRX Ref"=w190:T1)  [unwired: 7 in, 1 out]
          n77 = call <vilib>:"WPI_CANTalonSRX_ChangeMode.vi"("Output"=0.1, "Control Mode"=WPI_CANTalonSRX_APIControlMode."Percent VBus", "CAN Talon SRX Ref"=w200) -> ("CAN Talon SRX Ref"=w189:T1)  [unwired: 7 in, 1 out]
        }
        frame #4 {
          n78 = call <vilib>:"WPI_MotorControlSetOutput.vi"("Output"=-0.8, "MotorControlDevRef"=w241) -> ("MotorControlDevRef"=w240:T1)  [unwired: 7 in, 2 out]
          n79 = call-poly <vilib>:"WPI_RobotDriveArcadeDrive.vi"("Y axis value"=0.0, "X axis value"=0.0, "RobotDriveDevRef"=w230) -> ("error out"=w234:errorcluster, "RobotDriveDevRef"=w229:T14)  [unwired: 6 in, 1 out]
          n80 = call <vilib>:"WPI_RobotDriveDelayAndUpdateSafety.vi"("error in (no error)"=w234, "Delay (s)"=2.0, "RobotDriveDevRef"=w229) -> ("RobotDriveDevRef 2"=w228:T14)  [unwired: 7 in, 1 out]
          n81 = call <vilib>:"WPI_CANTalonSRX_SetReference.vi"("Reverse Closed-Loop Output"=TRUE, "Feedback Reference"=WPI_CANTalonSRX_APIFeedbackSelect."Count on Quad-A (Rising-Edge)", "CAN Talon SRX Ref"=w236) -> ("CAN Talon SRX Ref"=w265:T1)  [unwired: 7 in, 1 out]
          n82 = call <vilib>:"WPI_CANTalonSRX_SetReference.vi"("Feedback Reference"=WPI_CANTalonSRX_APIFeedbackSelect."Count on Quad-A (Rising-Edge)", "CAN Talon SRX Ref"=w238) -> ("CAN Talon SRX Ref"=w253:T1)  [unwired: 8 in, 1 out]
          n83 = call-poly <vilib>:"NT Read Value.vi"("Name"="Top P") -> ("Numeric"=w258:dbl)  [unwired: 9 in, 1 out]
          n84 = call-poly <vilib>:"NT Read Value.vi"("Name"="Top I") -> ("Numeric"=w257:dbl)  [unwired: 9 in, 1 out]
          n85 = call-poly <vilib>:"NT Read Value.vi"("Name"="Bottom P") -> ("Numeric"=w246:dbl)  [unwired: 9 in, 1 out]
          n86 = call-poly <vilib>:"NT Read Value.vi"("Name"="Bottom I") -> ("Numeric"=w245:dbl)  [unwired: 9 in, 1 out]
          n87 = call-poly <vilib>:"NT Read Value.vi"("Name"="Top D") -> ("Numeric"=w256:dbl)  [unwired: 9 in, 1 out]
          n88 = call <vilib>:"WPI_CANTalonSRX_SetPID.vi"("CAN Talon SRX Ref"=w265, "P"=w258, "I"=w257, "D"=w256, "F"=0.0) -> ("CAN Talon SRX Ref"=w263:T1)  [unwired: 9 in, 1 out]
          n89 = call-poly <vilib>:"NT Read Value.vi"("Name"="Bottom D") -> ("Numeric"=w244:dbl)  [unwired: 9 in, 1 out]
          n90 = call <vilib>:"WPI_CANTalonSRX_SetPID.vi"("CAN Talon SRX Ref"=w253, "P"=w246, "I"=w245, "D"=w244, "F"=0.0) -> ("CAN Talon SRX Ref"=w251:T1)  [unwired: 9 in, 1 out]
          n91 = call <vilib>:"WPI_CANTalonSRX_ChangeMode.vi"("Output"=0.7, "Control Mode"=WPI_CANTalonSRX_APIControlMode."Percent VBus", "CAN Talon SRX Ref"=w263) -> ("CAN Talon SRX Ref"=w235:T1)  [unwired: 7 in, 1 out]
          n92 = call <vilib>:"WPI_CANTalonSRX_ChangeMode.vi"("Output"=0.1, "Control Mode"=WPI_CANTalonSRX_APIControlMode."Percent VBus", "CAN Talon SRX Ref"=w251) -> ("CAN Talon SRX Ref"=w239:T1)  [unwired: 7 in, 1 out]
        }
        frame #5 {
          n93 = call-poly <vilib>:"WPI_RobotDriveArcadeDrive.vi"("Y axis value"=0.0, "X axis value"=0.0, "RobotDriveDevRef"=w271) -> ()  [unwired: 6 in, 3 out]
          n94 = call <vilib>:"WPI_MotorControlSetOutput.vi"("Output"=0.0, "MotorControlDevRef"=w268) -> ()  [unwired: 7 in, 3 out]
          n95 = call <vilib>:"WPI_MotorControlSetOutput.vi"("Output"=0.0, "MotorControlDevRef"=w267) -> ()  [unwired: 7 in, 3 out]
          n96 = call <vilib>:"WPI_MotorControlSetOutput.vi"("Output"=0.0, "MotorControlDevRef"=w275) -> ()  [unwired: 7 in, 3 out]
          n97 = call <vilib>:"WPI_CANTalonSRX_SetReference.vi"("Reverse Closed-Loop Output"=TRUE, "Feedback Reference"=WPI_CANTalonSRX_APIFeedbackSelect."Count on Quad-A (Rising-Edge)", "CAN Talon SRX Ref"=w277) -> ("CAN Talon SRX Ref"=w301:T1)  [unwired: 7 in, 1 out]
          n98 = call <vilib>:"WPI_CANTalonSRX_SetReference.vi"("Feedback Reference"=WPI_CANTalonSRX_APIFeedbackSelect."Count on Quad-A (Rising-Edge)", "CAN Talon SRX Ref"=w274) -> ("CAN Talon SRX Ref"=w289:T1)  [unwired: 8 in, 1 out]
          n99 = call-poly <vilib>:"NT Read Value.vi"("Name"="Top P") -> ("Numeric"=w294:dbl)  [unwired: 9 in, 1 out]
          n100 = call-poly <vilib>:"NT Read Value.vi"("Name"="Top I") -> ("Numeric"=w293:dbl)  [unwired: 9 in, 1 out]
          n101 = call-poly <vilib>:"NT Read Value.vi"("Name"="Bottom P") -> ("Numeric"=w282:dbl)  [unwired: 9 in, 1 out]
          n102 = call-poly <vilib>:"NT Read Value.vi"("Name"="Bottom I") -> ("Numeric"=w281:dbl)  [unwired: 9 in, 1 out]
          n103 = call-poly <vilib>:"NT Read Value.vi"("Name"="Top D") -> ("Numeric"=w292:dbl)  [unwired: 9 in, 1 out]
          n104 = call <vilib>:"WPI_CANTalonSRX_SetPID.vi"("CAN Talon SRX Ref"=w301, "P"=w294, "I"=w293, "D"=w292, "F"=0.0) -> ("CAN Talon SRX Ref"=w299:T1)  [unwired: 9 in, 1 out]
          n105 = call-poly <vilib>:"NT Read Value.vi"("Name"="Bottom D") -> ("Numeric"=w280:dbl)  [unwired: 9 in, 1 out]
          n106 = call <vilib>:"WPI_CANTalonSRX_SetPID.vi"("CAN Talon SRX Ref"=w289, "P"=w282, "I"=w281, "D"=w280, "F"=0.0) -> ("CAN Talon SRX Ref"=w287:T1)  [unwired: 9 in, 1 out]
          n107 = call <vilib>:"WPI_CANTalonSRX_ChangeMode.vi"("Output"=0.0, "Control Mode"=WPI_CANTalonSRX_APIControlMode."Percent VBus", "CAN Talon SRX Ref"=w299) -> ()  [unwired: 7 in, 2 out]
          n108 = call <vilib>:"WPI_CANTalonSRX_ChangeMode.vi"("Output"=0.0, "Control Mode"=WPI_CANTalonSRX_APIControlMode."Percent VBus", "CAN Talon SRX Ref"=w287) -> ()  [unwired: 7 in, 2 out]
        }
      }
    }
    frame 9 {
      # "portcullis"
      n109 = flat-sequence {
        tunnel: w314 -> [w334]
        tunnel: w315 -> [w329]
        tunnel: w316 -> [w331]
        tunnel: w317 -> [w332]
        tunnel: [w328] -> w313
        tunnel: [w334] -> w312
        tunnel: [w333] -> w311
        tunnel: [w330] -> w310
        tunnel: w309 -> [w327]
        tunnel: w304 -> [w326]
        tunnel: [w326] -> w303
        tunnel: [w361] -> w325
        tunnel: [w360] -> w324
        tunnel: [w353] -> w323
        tunnel: [w355] -> w322
        tunnel: [w359] -> w321
        tunnel: w313 -> [w354]
        tunnel: w312 -> [w352]
        tunnel: w311 -> [w358]
        tunnel: w310 -> [w356]
        tunnel: [w352] -> w308
        tunnel: w307 -> [w350]
        tunnel: [w349] -> w306
        tunnel: w305 -> [w348]
        tunnel: w303 -> [w347]
        tunnel: [w401] -> w320
        tunnel: [w400] -> w319
        tunnel: [w399] -> w318
        tunnel: w321 -> [w395]
        tunnel: w322 -> [w396]
        tunnel: w323 -> [w394]
        tunnel: w324 -> [w398]
        tunnel: w325 -> [w397]
        tunnel: w308 -> [w393]
        tunnel: w306 -> [w390]
        tunnel: w320 -> [w449]
        tunnel: w319 -> [w448]
        tunnel: w318 -> [w447]
        frame #0 {
          n110 = while {
            tunnel: [w341] -> w333
            tunnel: [w340] -> w328
            tunnel: [w339] -> w330
            tunnel: w332 -> [w338]
            tunnel: w331 -> [w337]
            tunnel: w329 -> [w336]
            tunnel: w327 -> [w335]
            stop <- w342 stop-if-true
            n111 = call <vilib>:"WPI_SwitchGetLimitValue.vi"("SwitchDevRef"=w335) -> ("Switch Pressed"=w342:bool)  [unwired: 8 in, 2 out]
            n112 = call <vilib>:"WPI_MotorControlSetOutput.vi"("Output"=0.4, "MotorControlDevRef"=w336) -> ("MotorControlDevRef"=w340:T1)  [unwired: 7 in, 2 out]
            n113 = call <vilib>:"WPI_MotorControlSetOutput.vi"("Output"=-0.4, "MotorControlDevRef"=w337) -> ("MotorControlDevRef"=w339:T1)  [unwired: 7 in, 2 out]
            n114 = call <vilib>:"WPI_RobotDriveTankDrive.vi"("Right axis value"=0.0, "Left axis value"=0.0, "RobotDriveDevRef"=w338) -> ("RobotDriveDevRef"=w341:T14)  [unwired: 6 in, 2 out]
          }
        }
        frame #1 {
          n115 = while {
            tunnel: w358 -> [w387]
            tunnel: [w383] -> w361
            tunnel: [w382] -> w360
            tunnel: [w381] -> w359
            tunnel: w350 -> [w367]
            tunnel: [w366] -> w349
            tunnel: w348 -> [w365]
            tunnel: w347 -> [w364]
            stop <- w384 stop-if-true
            n116 = call <vilib>:"WPI_GyroGetAngle.vi"("GyroDevRef"=w367) -> ("Angle"=w369:dbl, "GyroDevRef"=w366:T11)  [unwired: 6 in, 3 out]
            n117 = Greater?(x=w369, y=0.5) -> (0:w375:bool)
            n118 = Less?(x=w369, y=-0.5) -> (x < y?=w371:bool)
            n119 = Select(t=-0.7, s=w375, f=-0.65) -> (s? t:f=w363:dbl)
            n120 = call-poly <vilib>:"NT Read Value.vi"("Name"="First Drive") -> ("Numeric"=w380:dbl)  [unwired: 9 in, 1 out]
            n121 = call <vilib>:"WPI_EncoderGet.vi"("EncoderDevRef"=w365) -> ("Distance"=w389:dbl, "EncoderDevRef"=w383:T15)  [unwired: 5 in, 4 out]
            n122 = call <vilib>:"WPI_EncoderGet.vi"("EncoderDevRef"=w364) -> ("Distance"=w388:dbl, "EncoderDevRef"=w382:T15)  [unwired: 5 in, 4 out]
            n123 = Select(t=-0.7, s=w371, f=-0.65) -> (s? t:f=w362:dbl)
            n124 = call <vilib>:"WPI_RobotDriveTankDrive.vi"("Right axis value"=w363, "Left axis value"=w362, "RobotDriveDevRef"=w387) -> ("RobotDriveDevRef"=w381:T14)  [unwired: 6 in, 2 out]
            n125 = Absolute Value(x=w389) -> (abs(x)=w378:dbl)
            n126 = Absolute Value(x=w388) -> (abs(x)=w377:dbl)
            n127 = Greater?(x=w378, y=w380) -> (0:w386:bool)
            n128 = Greater?(x=w377, y=w380) -> (0:w385:bool)
            n129 = Or(x=w386, y=w385) -> (x .or. y?=w384:bool)
          }
          n130 = call <vilib>:"WPI_MotorControlSetOutput.vi"("Output"=0.0, "MotorControlDevRef"=w356) -> ("MotorControlDevRef"=w355:T1)  [unwired: 7 in, 2 out]
          n131 = call <vilib>:"WPI_MotorControlSetOutput.vi"("Output"=0.0, "MotorControlDevRef"=w354) -> ("MotorControlDevRef"=w353:T1)  [unwired: 7 in, 2 out]
        }
        frame #2 {
          n132 = call <vilib>:"WPI_EncoderReset.vi"("EncoderDevRef"=w398) -> ("EncoderDevRef"=w391:T15)  [unwired: 9 in, 1 out]
          n133 = call <vilib>:"WPI_EncoderReset.vi"("EncoderDevRef"=w397) -> ("EncoderDevRef"=w392:T15)  [unwired: 9 in, 1 out]
          n134 = while {
            tunnel: [w430] -> _
            tunnel: [w429] -> w399
            tunnel: w395 -> [w428]
            tunnel: [w419] -> _
            tunnel: [w427] -> _
            tunnel: [w425] -> w401
            tunnel: [w424] -> w400
            tunnel: w391 -> [w423]
            tunnel: w392 -> [w422]
            tunnel: w394 -> [w418]
            tunnel: w396 -> [w419]
            tunnel: w393 -> [w416]
            tunnel: w390 -> [w404]
            stop <- w426 stop-if-true
            n135 = call <vilib>:"WPI_GyroGetAngle.vi"("GyroDevRef"=w404) -> ("Angle"=w406:dbl)  [unwired: 6 in, 4 out]
            n136 = Greater?(x=w406, y=0.5) -> (0:w412:bool)
            n137 = Less?(x=w406, y=-0.5) -> (x < y?=w408:bool)
            n138 = Select(t=-0.7, s=w412, f=-0.65) -> (s? t:f=w402:dbl)
            n139 = Select(t=-0.7, s=w408, f=-0.65) -> (s? t:f=w403:dbl)
            n140 = call <vilib>:"WPI_RobotDriveTankDrive.vi"("Right axis value"=w402, "Left axis value"=w403, "RobotDriveDevRef"=w428) -> ("RobotDriveDevRef"=w429:T14)  [unwired: 6 in, 2 out]
            n141 = call-poly <vilib>:"NT Read Value.vi"("Name"="Second Drive") -> ("Numeric"=w420:dbl)  [unwired: 9 in, 1 out]
            n142 = call <vilib>:"WPI_EncoderGet.vi"("EncoderDevRef"=w422) -> ("Distance"=w434:dbl, "EncoderDevRef"=w427:T15)  [unwired: 5 in, 4 out]
            n143 = call <vilib>:"WPI_EncoderGet.vi"("EncoderDevRef"=w423) -> ("Distance"=w433:dbl, "EncoderDevRef"=w430:T15)  [unwired: 5 in, 4 out]
            n144 = call <vilib>:"WPI_SwitchGetLimitValue.vi"("SwitchDevRef"=w416) -> ("Switch Pressed"=w417:bool)  [unwired: 8 in, 2 out]
            n145 = Absolute Value(x=w434) -> (abs(x)=w415:dbl)
            n146 = Absolute Value(x=w433) -> (abs(x)=w414:dbl)
            n147 = case shown="False" w417 {
              tunnel: w419 -> [w436 w444]
              tunnel: [w437 w443] -> w425
              tunnel: [w438 w442] -> w424
              tunnel: w418 -> [w435 w441]
              frame False {
                # "If switch is not pressed\nmove motors up until pressed"
                n148 = call <vilib>:"WPI_MotorControlSetOutput.vi"("Output"=-0.4, "MotorControlDevRef"=w435) -> ("MotorControlDevRef"=w437:T1)  [unwired: 7 in, 2 out]
                n149 = call <vilib>:"WPI_MotorControlSetOutput.vi"("Output"=0.4, "MotorControlDevRef"=w436) -> ("MotorControlDevRef"=w438:T1)  [unwired: 7 in, 2 out]
              }
              frame True {
                # "If switch is pressed, stop motors"
                n150 = call <vilib>:"WPI_MotorControlSetOutput.vi"("Output"=0.0, "MotorControlDevRef"=w444) -> ("MotorControlDevRef"=w443:T1)  [unwired: 7 in, 2 out]
                n151 = call <vilib>:"WPI_MotorControlSetOutput.vi"("Output"=0.0, "MotorControlDevRef"=w441) -> ("MotorControlDevRef"=w442:T1)  [unwired: 7 in, 2 out]
              }
            }
            n152 = Greater?(x=w415, y=w420) -> (0:w432:bool)
            n153 = Greater?(x=w414, y=w420) -> (0:w431:bool)
            n154 = Or(x=w432, y=w431) -> (x .or. y?=w426:bool)
          }
        }
        frame #3 {
          n155 = call <vilib>:"WPI_RobotDriveTankDrive.vi"("Right axis value"=0.0, "Left axis value"=0.0, "RobotDriveDevRef"=w447) -> ()  [unwired: 6 in, 3 out]
          n156 = call <vilib>:"WPI_MotorControlSetOutput.vi"("Output"=0.0, "MotorControlDevRef"=w449) -> ()  [unwired: 7 in, 3 out]
          n157 = call <vilib>:"WPI_MotorControlSetOutput.vi"("Output"=0.0, "MotorControlDevRef"=w448) -> ()  [unwired: 7 in, 3 out]
        }
      }
    }
    frame 10 {
      # "cheval"
      n158 = flat-sequence {
        tunnel: w481 -> [w499]
        tunnel: [w498] -> w487
        tunnel: [w497] -> w486
        tunnel: [w496] -> w485
        tunnel: [w495] -> w480
        tunnel: w479 -> [w495]
        tunnel: [w494] -> w478
        tunnel: w477 -> [w494]
        tunnel: w476 -> [w493]
        tunnel: [w493] -> w475
        tunnel: [w492] -> w474
        tunnel: w473 -> [w492]
        tunnel: w460 -> [w491]
        tunnel: [w490] -> w458
        tunnel: w456 -> [w489]
        tunnel: w455 -> [w488]
        tunnel: [w544] -> w464
        tunnel: [w543] -> w466
        tunnel: [w532] -> w468
        tunnel: [w542] -> w470
        tunnel: [w541] -> w472
        tunnel: w480 -> [_]
        tunnel: w485 -> [w543]
        tunnel: w486 -> [w540]
        tunnel: w487 -> [w544]
        tunnel: w478 -> [w539]
        tunnel: w475 -> [w538]
        tunnel: [w537] -> w462
        tunnel: w474 -> [w537]
        tunnel: [w536] -> w459
        tunnel: w458 -> [w536]
        tunnel: w454 -> [w530]
        tunnel: w472 -> [w566]
        tunnel: [w566] -> w471
        tunnel: w470 -> [w565]
        tunnel: [w565] -> w469
        tunnel: w468 -> [w559]
        tunnel: [w559] -> w467
        tunnel: w466 -> [w563]
        tunnel: [w560] -> w465
        tunnel: w464 -> [w562]
        tunnel: [w561] -> w463
        tunnel: w462 -> [w564]
        tunnel: [w564] -> w461
        tunnel: w459 -> [w558]
        tunnel: [w557] -> w457
        tunnel: w471 -> [w601]
        tunnel: w469 -> [w600]
        tunnel: w467 -> [w602]
        tunnel: w465 -> [w596]
        tunnel: w463 -> [w595]
        tunnel: [w599] -> w484
        tunnel: [w598] -> w483
        tunnel: [w597] -> w482
        tunnel: w461 -> [w594]
        tunnel: w457 -> [w591]
        tunnel: w484 -> [w650]
        tunnel: w483 -> [w649]
        tunnel: w482 -> [w648]
        frame #0 {
          n159 = while {
            tunnel: w499 -> [w525]
            tunnel: [w521] -> w498
            tunnel: [w520] -> w496
            tunnel: [w519] -> w497
            tunnel: w491 -> [w505]
            tunnel: [w504] -> w490
            tunnel: w489 -> [w503]
            tunnel: w488 -> [w502]
            stop <- w522 stop-if-true
            n160 = call <vilib>:"WPI_GyroGetAngle.vi"("GyroDevRef"=w505) -> ("Angle"=w508:dbl, "GyroDevRef"=w504:T11)  [unwired: 6 in, 3 out]
            n161 = call-poly <vilib>:"NT Read Value.vi"("Name"="First Drive") -> ("Numeric"=w518:dbl)  [unwired: 9 in, 1 out]
            n162 = call <vilib>:"WPI_EncoderGet.vi"("EncoderDevRef"=w503) -> ("Distance"=w527:dbl, "EncoderDevRef"=w521:T15)  [unwired: 5 in, 4 out]
            n163 = call <vilib>:"WPI_EncoderGet.vi"("EncoderDevRef"=w502) -> ("Distance"=w526:dbl, "EncoderDevRef"=w520:T15)  [unwired: 5 in, 4 out]
            n164 = Greater?(x=w508, y=0.5) -> (0:w513:bool)
            n165 = Less?(x=w508, y=-0.5) -> (x < y?=w510:bool)
            n166 = Absolute Value(x=w526) -> (abs(x)=w515:dbl)
            n167 = Absolute Value(x=w527) -> (abs(x)=w516:dbl)
            n168 = Greater?(x=w516, y=w518) -> (0:w524:bool)
            n169 = Greater?(x=w515, y=w518) -> (0:w523:bool)
            n170 = Select(t=-0.7, s=w513, f=-0.65) -> (s? t:f=w501:dbl)
            n171 = Select(t=-0.7, s=w510, f=-0.65) -> (s? t:f=w500:dbl)
            n172 = call <vilib>:"WPI_RobotDriveTankDrive.vi"("Right axis value"=w501, "Left axis value"=w500, "RobotDriveDevRef"=w525) -> ("RobotDriveDevRef"=w519:T14)  [unwired: 6 in, 2 out]
            n173 = Or(x=w524, y=w523) -> (x .or. y?=w522:bool)
          }
        }
        frame #1 {
          n174 = call <vilib>:"WPI_SwitchGetLimitValue.vi"("SwitchDevRef"=w530) -> ("Switch Pressed"=w529:bool)  [unwired: 8 in, 2 out]
          n175 = Not(x=w529) -> (.not. x?=w528:bool)
          n176 = case shown="False" w528 {
            tunnel: [w546 w556] -> w542
            tunnel: [w545 w555] -> w541
            tunnel: w539 -> [w547 w554]
            tunnel: w538 -> [w548 w553]
            frame False {
              n177 = call <vilib>:"WPI_MotorControlSetOutput.vi"("Output"=0.0, "MotorControlDevRef"=w547) -> ("MotorControlDevRef"=w545:T1)  [unwired: 7 in, 2 out]
              n178 = call <vilib>:"WPI_MotorControlSetOutput.vi"("Output"=0.0, "MotorControlDevRef"=w548) -> ("MotorControlDevRef"=w546:T1)  [unwired: 7 in, 2 out]
            }
            frame True {
              n179 = call <vilib>:"WPI_MotorControlSetOutput.vi"("Output"=-0.4, "MotorControlDevRef"=w554) -> ("MotorControlDevRef"=w555:T1)  [unwired: 7 in, 2 out]
              n180 = call <vilib>:"WPI_MotorControlSetOutput.vi"("Output"=0.4, "MotorControlDevRef"=w553) -> ("MotorControlDevRef"=w556:T1)  [unwired: 7 in, 2 out]
            }
          }
          n181 = call <vilib>:"WPI_RobotDriveTankDrive.vi"("Right axis value"=0.0, "Left axis value"=0.0, "RobotDriveDevRef"=w540) -> ("RobotDriveDevRef"=w533:T14)  [unwired: 6 in, 2 out]
          n182 = call <vilib>:"WPI_RobotDriveDelayAndUpdateSafety.vi"("Delay (s)"=3.0, "RobotDriveDevRef"=w533) -> ("RobotDriveDevRef 2"=w532:T14)  [unwired: 8 in, 1 out]
        }
        frame #2 {
          n183 = call <vilib>:"WPI_EncoderReset.vi"("EncoderDevRef"=w563) -> ("EncoderDevRef"=w560:T15)  [unwired: 9 in, 1 out]
          n184 = call <vilib>:"WPI_EncoderReset.vi"("EncoderDevRef"=w562) -> ("EncoderDevRef"=w561:T15)  [unwired: 9 in, 1 out]
          n185 = while {
            tunnel: w560 -> [w588]
            tunnel: w561 -> [w587]
            tunnel: w559 -> [w582]
            tunnel: w558 -> [w570]
            tunnel: [w569] -> w557
            stop <- w584 stop-if-true
            w583 = -1.0 ("y")
            n186 = call <vilib>:"WPI_GyroGetAngle.vi"("GyroDevRef"=w570) -> ("Angle"=w573:dbl, "GyroDevRef"=w569:T11)  [unwired: 6 in, 3 out]
            n187 = Greater?(x=w573, y=0.5) -> (0:w578:bool)
            n188 = Less?(x=w573, y=-0.5) -> (x < y?=w575:bool)
            n189 = call <vilib>:"WPI_EncoderGet.vi"("EncoderDevRef"=w588) -> ("Distance"=w589:dbl)  [unwired: 5 in, 5 out]
            n190 = call <vilib>:"WPI_EncoderGet.vi"("EncoderDevRef"=w587) -> ("Distance"=w590:dbl)  [unwired: 5 in, 5 out]
            n191 = Select(t=0.95, s=w578, f=0.9) -> (s? t:f=w567:dbl)
            n192 = Absolute Value(x=w589) -> (abs(x)=w581:dbl)
            n193 = Select(t=0.95, s=w575, f=0.7) -> (s? t:f=w568:dbl)
            n194 = call <vilib>:"WPI_RobotDriveTankDrive.vi"("Right axis value"=w567, "Left axis value"=w568, "RobotDriveDevRef"=w582) -> ()  [unwired: 6 in, 3 out]
            n195 = Absolute Value(x=w590) -> (abs(x)=w580:dbl)
            n196 = Greater?(x=w581, y=w583) -> (0:w586:bool)
            n197 = Greater?(x=w580, y=w583) -> (0:w585:bool)
            n198 = Or(x=w586, y=w585) -> (x .or. y?=w584:bool)
          }
        }
        frame #3 {
          n199 = call <vilib>:"WPI_EncoderReset.vi"("EncoderDevRef"=w596) -> ("EncoderDevRef"=w592:T15)  [unwired: 9 in, 1 out]
          n200 = call <vilib>:"WPI_EncoderReset.vi"("EncoderDevRef"=w595) -> ("EncoderDevRef"=w593:T15)  [unwired: 9 in, 1 out]
          n201 = while {
            tunnel: [w631] -> _
            tunnel: [w630] -> w597
            tunnel: w602 -> [w629]
            tunnel: w601 -> [w626]
            tunnel: w600 -> [w625]
            tunnel: [w628] -> _
            tunnel: [w623] -> w599
            tunnel: [w622] -> w598
            tunnel: w592 -> [w621]
            tunnel: w593 -> [w620]
            tunnel: w594 -> [w617]
            tunnel: w591 -> [w605]
            stop <- w624 stop-if-true
            n202 = call <vilib>:"WPI_SwitchGetLimitValue.vi"("SwitchDevRef"=w617) -> ("Switch Pressed"=w627:bool)  [unwired: 8 in, 2 out]
            n203 = case shown="True" w627 {
              tunnel: w626 -> [w639 w645]
              tunnel: w625 -> [w638 w644]
              tunnel: [w636 w643] -> w623
              tunnel: [w637 w642] -> w622
              frame False {
                # "If switch is not pressed\nmove motors up until pressed"
                n204 = call <vilib>:"WPI_MotorControlSetOutput.vi"("Output"=-0.4, "MotorControlDevRef"=w638) -> ("MotorControlDevRef"=w636:T1)  [unwired: 7 in, 2 out]
                n205 = call <vilib>:"WPI_MotorControlSetOutput.vi"("Output"=0.4, "MotorControlDevRef"=w639) -> ("MotorControlDevRef"=w637:T1)  [unwired: 7 in, 2 out]
              }
              frame True {
                # "If switch is pressed, stop motors"
                n206 = call <vilib>:"WPI_MotorControlSetOutput.vi"("Output"=0.0, "MotorControlDevRef"=w644) -> ("MotorControlDevRef"=w643:T1)  [unwired: 7 in, 2 out]
                n207 = call <vilib>:"WPI_MotorControlSetOutput.vi"("Output"=0.0, "MotorControlDevRef"=w645) -> ("MotorControlDevRef"=w642:T1)  [unwired: 7 in, 2 out]
              }
            }
            n208 = call-poly <vilib>:"NT Read Value.vi"("Name"="Second Drive") -> ("Numeric"=w618:dbl)  [unwired: 9 in, 1 out]
            n209 = call <vilib>:"WPI_EncoderGet.vi"("EncoderDevRef"=w620) -> ("Distance"=w635:dbl, "EncoderDevRef"=w628:T15)  [unwired: 5 in, 4 out]
            n210 = call <vilib>:"WPI_EncoderGet.vi"("EncoderDevRef"=w621) -> ("Distance"=w634:dbl, "EncoderDevRef"=w631:T15)  [unwired: 5 in, 4 out]
            n211 = Absolute Value(x=w618) -> (abs(x)=w615:dbl)
            n212 = Absolute Value(x=w635) -> (abs(x)=w616:dbl)
            n213 = Greater?(x=w616, y=w615) -> (0:w633:bool)
            n214 = Greater?(x=w634, y=w615) -> (0:w632:bool)
            n215 = Or(x=w633, y=w632) -> (x .or. y?=w624:bool)
            n216 = call <vilib>:"WPI_GyroGetAngle.vi"("GyroDevRef"=w605) -> ("Angle"=w608:dbl)  [unwired: 6 in, 4 out]
            n217 = Greater?(x=w608, y=0.5) -> (0:w613:bool)
            n218 = Less?(x=w608, y=-0.5) -> (x < y?=w610:bool)
            n219 = Select(t=-0.95, s=w613, f=-0.9) -> (s? t:f=w603:dbl)
            n220 = Select(t=-0.95, s=w610, f=-0.9) -> (s? t:f=w604:dbl)
            n221 = call <vilib>:"WPI_RobotDriveTankDrive.vi"("Right axis value"=w603, "Left axis value"=w604, "RobotDriveDevRef"=w629) -> ("RobotDriveDevRef"=w630:T14)  [unwired: 6 in, 2 out]
          }
        }
        frame #4 {
          n222 = call <vilib>:"WPI_RobotDriveTankDrive.vi"("Right axis value"=0.0, "Left axis value"=0.0, "RobotDriveDevRef"=w648) -> ()  [unwired: 6 in, 3 out]
          n223 = call <vilib>:"WPI_MotorControlSetOutput.vi"("Output"=0.0, "MotorControlDevRef"=w650) -> ()  [unwired: 7 in, 3 out]
          n224 = call <vilib>:"WPI_MotorControlSetOutput.vi"("Output"=0.0, "MotorControlDevRef"=w649) -> ()  [unwired: 7 in, 3 out]
        }
      }
    }
    frame 8 {
      # "Just touching obsicle"
      n225 = flat-sequence {
        tunnel: w658 -> [w662]
        tunnel: [w661] -> w657
        tunnel: w656 -> [w660]
        tunnel: w655 -> [w659]
        tunnel: w657 -> [w675]
        frame #0 {
          n226 = while {
            tunnel: w662 -> [w666]
            tunnel: [w665] -> w661
            tunnel: w660 -> [w664]
            tunnel: w659 -> [w663]
            stop <- w667 stop-if-true
            w669 = 36.0 ("y")
            n227 = call <vilib>:"WPI_EncoderGet.vi"("EncoderDevRef"=w664) -> ("Distance"=w672:dbl)  [unwired: 5 in, 5 out]
            n228 = call <vilib>:"WPI_EncoderGet.vi"("EncoderDevRef"=w663) -> ("Distance"=w670:dbl)  [unwired: 5 in, 5 out]
            n229 = call <vilib>:"WPI_RobotDriveTankDrive.vi"("Right axis value"=-0.65 ("Y axis value"), "Left axis value"=-0.65 ("X axis value"), "RobotDriveDevRef"=w666) -> ("RobotDriveDevRef"=w665:T14)  [unwired: 6 in, 2 out]
            n230 = Greater?(x=w672, y=w669) -> (0:w671:bool)
            n231 = Greater?(x=w670, y=w669) -> (0:w668:bool)
            n232 = Or(x=w671, y=w668) -> (x .or. y?=w667:bool)
          }
        }
        frame #1 {
          n233 = call-poly <vilib>:"WPI_RobotDriveArcadeDrive.vi"("Y axis value"=0.0, "X axis value"=0.0, "RobotDriveDevRef"=w675) -> ()  [unwired: 6 in, 3 out]
        }
      }
    }
    frame 2 {
      # "One ball autonomus from behind low bar to high goal"
      n234 = flat-sequence {
        tunnel: [w763] -> w724
        tunnel: [w762] -> w723
        tunnel: [w761] -> w722
        tunnel: [w760] -> w721
        tunnel: [w759] -> w720
        tunnel: [w758] -> w719
        tunnel: w749 -> [w757]
        tunnel: w748 -> [w763]
        tunnel: w747 -> [w762]
        tunnel: w746 -> [w761]
        tunnel: w734 -> [w760]
        tunnel: w733 -> [w759]
        tunnel: w732 -> [w758]
        tunnel: w725 -> [w756]
        tunnel: [w755] -> w718
        tunnel: [w754] -> w717
        tunnel: [w753] -> w716
        tunnel: [w752] -> w715
        tunnel: w713 -> [w751]
        tunnel: w712 -> [w750]
        tunnel: w724 -> [w803]
        tunnel: [w803] -> w711
        tunnel: w723 -> [w802]
        tunnel: [w802] -> w709
        tunnel: w722 -> [w801]
        tunnel: [w801] -> w707
        tunnel: [w792] -> w705
        tunnel: [w800] -> w703
        tunnel: w721 -> [w800]
        tunnel: w720 -> [w799]
        tunnel: [w799] -> w701
        tunnel: [w798] -> w699
        tunnel: w719 -> [w798]
        tunnel: w718 -> [w797]
        tunnel: [w796] -> w697
        tunnel: w717 -> [w796]
        tunnel: [w795] -> w695
        tunnel: w716 -> [w795]
        tunnel: [w793] -> w693
        tunnel: w715 -> [w794]
        tunnel: w711 -> [w829]
        tunnel: [w829] -> w710
        tunnel: w709 -> [w828]
        tunnel: [w828] -> w708
        tunnel: w707 -> [w827]
        tunnel: [w827] -> w706
        tunnel: w705 -> [w817]
        tunnel: [w814] -> w704
        tunnel: w703 -> [w826]
        tunnel: [w826] -> w702
        tunnel: w701 -> [w825]
        tunnel: [w825] -> w700
        tunnel: w699 -> [w824]
        tunnel: [w824] -> w698
        tunnel: w697 -> [w823]
        tunnel: [w823] -> w696
        tunnel: w695 -> [w822]
        tunnel: [w822] -> w694
        tunnel: w693 -> [w821]
        tunnel: [w821] -> w692
        tunnel: w710 -> [w842]
        tunnel: [w842] -> w691
        tunnel: w708 -> [w841]
        tunnel: [w841] -> w689
        tunnel: w706 -> [w840]
        tunnel: [w840] -> w687
        tunnel: w704 -> [w839]
        tunnel: [w838] -> w685
        tunnel: [w835] -> w684
        tunnel: w702 -> [w835]
        tunnel: w700 -> [w834]
        tunnel: [w834] -> w682
        tunnel: [w833] -> w680
        tunnel: w698 -> [w833]
        tunnel: w696 -> [w832]
        tunnel: w694 -> [w831]
        tunnel: w692 -> [w830]
        tunnel: w691 -> [w883]
        tunnel: [w883] -> w690
        tunnel: w689 -> [w882]
        tunnel: [w882] -> w688
        tunnel: w687 -> [w881]
        tunnel: [w881] -> w686
        tunnel: w685 -> [w875]
        tunnel: w684 -> [w880]
        tunnel: [w880] -> w683
        tunnel: w682 -> [w879]
        tunnel: [w879] -> w681
        tunnel: w680 -> [w878]
        tunnel: [w878] -> w679
        tunnel: [w874] -> w678
        tunnel: w690 -> [w915]
        tunnel: [w915] -> w737
        tunnel: w688 -> [w914]
        tunnel: [w914] -> w736
        tunnel: w686 -> [w913]
        tunnel: [w913] -> w735
        tunnel: w683 -> [w912]
        tunnel: w681 -> [w910]
        tunnel: w679 -> [w911]
        tunnel: [w909] -> w731
        tunnel: [w908] -> w730
        tunnel: [w907] -> w714
        tunnel: w678 -> [w906]
        tunnel: [w977] -> w745
        tunnel: w737 -> [w941]
        tunnel: w736 -> [_]
        tunnel: w735 -> [_]
        tunnel: [w944] -> w744
        tunnel: [w943] -> w742
        tunnel: [w940] -> w739
        tunnel: w731 -> [w937]
        tunnel: w730 -> [w936]
        tunnel: [w935] -> w728
        tunnel: [w934] -> w727
        tunnel: w714 -> [w928]
        tunnel: w745 -> [w997]
        tunnel: w744 -> [w993]
        tunnel: [w992] -> w743
        tunnel: w742 -> [w994]
        tunnel: [w996] -> w741
        tunnel: [w995] -> w740
        tunnel: w739 -> [w987]
        tunnel: [w985] -> w738
        tunnel: [w984] -> w729
        tunnel: w728 -> [w984]
        tunnel: w727 -> [w983]
        tunnel: [w983] -> w726
        tunnel: w743 -> [w1032]
        tunnel: w741 -> [w1030]
        tunnel: w740 -> [w1029]
        tunnel: w738 -> [w1026]
        tunnel: w729 -> [w1024]
        tunnel: w726 -> [w1022]
        frame #0 {
          n235 = while {
            shift-right: [w790] -> w755
            shift-left: w757 -> [w791]
            tunnel: [w784] -> w753
            tunnel: [w783] -> w754
            tunnel: w756 -> [w769]
            tunnel: [w768] -> w752
            tunnel: w751 -> [w765]
            tunnel: w750 -> [w764]
            stop <- w785 stop-if-true
            n236 = call-poly <vilib>:"NT Read Value.vi"("Name"="First Drive") -> ("Numeric"=w780:dbl)  [unwired: 9 in, 1 out]
            n237 = call <vilib>:"WPI_EncoderGet.vi"("EncoderDevRef"=w765) -> ("Distance"=w787:dbl, "EncoderDevRef"=w783:T15)  [unwired: 5 in, 4 out]
            n238 = call <vilib>:"WPI_EncoderGet.vi"("EncoderDevRef"=w764) -> ("Distance"=w789:dbl, "EncoderDevRef"=w784:T15)  [unwired: 5 in, 4 out]
            n239 = Absolute Value(x=w787) -> (abs(x)=w782:dbl)
            n240 = Absolute Value(x=w789) -> (abs(x)=w781:dbl)
            n241 = Greater?(x=w782, y=w780) -> (0:w786:bool)
            n242 = call <vilib>:"WPI_GyroGetAngle.vi"("GyroDevRef"=w769) -> ("Angle"=w777:dbl, "GyroDevRef"=w768:T11)  [unwired: 6 in, 3 out]
            n243 = Greater?(x=w781, y=w780) -> (0:w788:bool)
            n244 = Or(x=w786, y=w788) -> (x .or. y?=w785:bool)
            n245 = Greater?(x=w777, y=0.5) -> (0:w771:bool)
            n246 = Less?(x=w777, y=-0.5) -> (x < y?=w775:bool)
            n247 = Select(t=-0.7, s=w771, f=-0.65) -> (s? t:f=w766:dbl)
            n248 = Select(t=-0.7, s=w775, f=-0.65) -> (s? t:f=w767:dbl)
            n249 = call <vilib>:"WPI_RobotDriveTankDrive.vi"("Right axis value"=w766, "Left axis value"=w767, "RobotDriveDevRef"=w791) -> ("RobotDriveDevRef"=w790:T14)  [unwired: 6 in, 2 out]
          }
        }
        frame #1 {
          n250 = while {
            shift-right: [w810] -> w792
            shift-left: w797 -> [w812]
            tunnel: w794 -> [w805]
            tunnel: [w804] -> w793
            stop <- w806 stop-if-true
            n251 = call <vilib>:"WPI_GyroGetAngle.vi"("GyroDevRef"=w805) -> ("Angle"=w809:dbl, "GyroDevRef"=w804:T11)  [unwired: 6 in, 3 out]
            n252 = call <vilib>:"WPI_RobotDriveTankDrive.vi"("Right axis value"=-0.3 ("Y axis value"), "Left axis value"=-0.6 ("X axis value"), "RobotDriveDevRef"=w812) -> ("RobotDriveDevRef"=w810:T14)  [unwired: 6 in, 2 out]
            n253 = call-poly <vilib>:"NT Read Value.vi"("Name"="First Turn") -> ("Numeric"=w807:dbl)  [unwired: 9 in, 1 out]
            n254 = Greater?(x=w809, y=w807) -> (0:w806:bool)
          }
        }
        frame #2 {
          n255 = call-poly <vilib>:"WPI_RobotDriveArcadeDrive.vi"("Y axis value"=0.0, "X axis value"=0.0, "RobotDriveDevRef"=w817) -> ("error out"=w820:errorcluster, "RobotDriveDevRef"=w816:T14)  [unwired: 6 in, 1 out]
          n256 = call <vilib>:"WPI_RobotDriveDelayAndUpdateSafety.vi"("error in (no error)"=w820, "Delay (s)"=2.0, "RobotDriveDevRef"=w816) -> ("RobotDriveDevRef 2"=w814:T14)  [unwired: 7 in, 1 out]
        }
        frame #3 {
          n257 = call <vilib>:"WPI_EncoderReset.vi"("EncoderDevRef"=w832) -> ("EncoderDevRef"=w836:T15)  [unwired: 9 in, 1 out]
          n258 = call <vilib>:"WPI_EncoderReset.vi"("EncoderDevRef"=w831) -> ("EncoderDevRef"=w837:T15)  [unwired: 9 in, 1 out]
          n259 = while {
            shift-right: [w869] -> w838
            shift-left: w839 -> [w870]
            tunnel: w836 -> [w865]
            tunnel: w837 -> [w860]
            tunnel: w830 -> [w851]
            stop <- w861 stop-if-true
            w847 = 0.5 ("y")
            n260 = call-poly <vilib>:"NT Read Value.vi"("Name"="Second Drive") -> ("Numeric"=w863:dbl)  [unwired: 9 in, 1 out]
            n261 = call-poly <vilib>:"NT Read Value.vi"("Name"="First Turn") -> ("Numeric"=w846:dbl)  [unwired: 9 in, 1 out]
            n262 = call <vilib>:"WPI_EncoderGet.vi"("EncoderDevRef"=w865) -> ("Distance"=w864:dbl)  [unwired: 5 in, 5 out]
            n263 = call <vilib>:"WPI_EncoderGet.vi"("EncoderDevRef"=w860) -> ("Distance"=w867:dbl)  [unwired: 5 in, 5 out]
            n264 = Absolute Value(x=w864) -> (abs(x)=w859:dbl)
            n265 = Absolute Value(x=w867) -> (abs(x)=w858:dbl)
            n266 = Greater?(x=w859, y=w863) -> (0:w862:bool)
            n267 = Greater?(x=w858, y=w863) -> (0:w866:bool)
            n268 = Or(x=w862, y=w866) -> (x .or. y?=w861:bool)
            n269 = Subtract(x=w846, y=w847) -> (x-y=w848:dbl)
            n270 = Add(x=w846, y=w847) -> (x+y=w845:dbl)
            n271 = call <vilib>:"WPI_GyroGetAngle.vi"("GyroDevRef"=w851) -> ("Angle"=w853:dbl)  [unwired: 6 in, 4 out]
            n272 = Less?(x=w853, y=w848) -> (x < y?=w855:bool)
            n273 = Greater?(x=w853, y=w845) -> (0:w857:bool)
            n274 = Select(t=-0.7, s=w855, f=-0.65) -> (s? t:f=w844:dbl)
            n275 = Select(t=-0.7, s=w857, f=-0.65) -> (s? t:f=w843:dbl)
            n276 = call <vilib>:"WPI_RobotDriveTankDrive.vi"("Right axis value"=w843, "Left axis value"=w844, "RobotDriveDevRef"=w870) -> ("RobotDriveDevRef"=w869:T14)  [unwired: 6 in, 2 out]
          }
        }
        frame #4 {
          n277 = call-poly <vilib>:"NT Read Value.vi"("Name"="X") -> ("Numeric"=w871:dbl)  [unwired: 9 in, 1 out]
          n278 = call-poly <vilib>:"NT Read Value.vi"("Name"="X Offset") -> ("Numeric"=w872:dbl)  [unwired: 9 in, 1 out]
          n279 = Greater?(x=w871, y=w872) -> (0:w873:bool)
          n280 = case shown="True" w873 {
            tunnel: w875 -> [w887 w898]
            tunnel: [w886 w897] -> w874
            tunnel: w871 -> [w885 _]
            tunnel: w872 -> [w884 w895]
            tunnel: w871 -> [_ w896]
            frame False {
              n281 = while {
                shift-right: [w891] -> w886
                shift-left: w887 -> [w892]
                tunnel: w885 -> [w890]
                tunnel: w884 -> [w889]
                stop <- w888 stop-if-true
                n282 = call <vilib>:"WPI_RobotDriveTankDrive.vi"("Right axis value"=0.6, "Left axis value"=-0.6, "RobotDriveDevRef"=w892) -> ("RobotDriveDevRef"=w891:T14)  [unwired: 6 in, 2 out]
                n283 = Greater Or Equal?(x=w890, y=w889) -> (x >= y?=w888:bool)
              }
            }
            frame True {
              n284 = while {
                shift-right: [w904] -> w897
                shift-left: w898 -> [w905]
                tunnel: w896 -> [w901]
                tunnel: w895 -> [w900]
                stop <- w899 stop-if-true
                n285 = call <vilib>:"WPI_RobotDriveTankDrive.vi"("Right axis value"=-0.6, "Left axis value"=0.6, "RobotDriveDevRef"=w905) -> ("RobotDriveDevRef"=w904:T14)  [unwired: 6 in, 2 out]
                n286 = Less Or Equal?(x=w901, y=w900) -> (x <= y?=w899:bool)
              }
            }
          }
        }
        frame #5 {
          n287 = while {
            tunnel: w912 -> [w921]
            tunnel: [w924] -> w909
            tunnel: [w923] -> w908
            tunnel: w911 -> [w922]
            tunnel: w910 -> [w920]
            tunnel: [w917] -> w907
            tunnel: w906 -> [w916]
            stop <- w925 stop-if-true
            n288 = call <vilib>:"WPI_MotorControlSetOutput.vi"("Output"=0.25, "MotorControlDevRef"=w920) -> ("MotorControlDevRef"=w924:T1)  [unwired: 7 in, 2 out]
            n289 = call <vilib>:"WPI_MotorControlSetOutput.vi"("Output"=-0.25, "MotorControlDevRef"=w921) -> ("MotorControlDevRef"=w923:T1)  [unwired: 7 in, 2 out]
            n290 = call <vilib>:"WPI_SwitchGetLimitValue.vi"("SwitchDevRef"=w922) -> ("Switch Pressed"=w925:bool)  [unwired: 8 in, 2 out]
            n291 = call <vilib>:"WPI_RobotDriveTankDrive.vi"("Right axis value"=0.0, "Left axis value"=0.0, "RobotDriveDevRef"=w916) -> ("RobotDriveDevRef"=w917:T14)  [unwired: 6 in, 2 out]
          }
        }
        frame #6 {
          n292 = call-poly <vilib>:"WPI_RobotDriveArcadeDrive.vi"("Y axis value"=0.0, "X axis value"=0.0, "RobotDriveDevRef"=w928) -> ("error out"=w975:errorcluster, "RobotDriveDevRef"=w974:T14)  [unwired: 6 in, 1 out]
          n293 = call <vilib>:"WPI_RobotDriveDelayAndUpdateSafety.vi"("error in (no error)"=w975, "Delay (s)"=3.0, "RobotDriveDevRef"=w974) -> ("RobotDriveDevRef 2"=w940:T14)  [unwired: 7 in, 1 out]
          n294 = call <vilib>:"WPI_MotorControlSetOutput.vi"("Output"=0.0, "MotorControlDevRef"=w937) -> ("MotorControlDevRef"=w935:T1)  [unwired: 7 in, 2 out]
          n295 = call <vilib>:"WPI_MotorControlSetOutput.vi"("Output"=0.0, "MotorControlDevRef"=w936) -> ("MotorControlDevRef"=w934:T1)  [unwired: 7 in, 2 out]
          n296 = call <vilib>:"WPI_MotorControlSetOutput.vi"("Output"=0.0, "MotorControlDevRef"=w941) -> ("MotorControlDevRef"=w977:T1)  [unwired: 7 in, 2 out]
          n297 = call <vilib>:"WPI_MotorControlRefNum Registry Get.vi"("refnum name"="Top Shooter") -> ("MotorControlDevRef"=w969:T1)  [unwired: 9 in, 1 out]
          n298 = call <vilib>:"WPI_MotorControlRefNum Registry Get.vi"("refnum name"="Bottom Shooter") -> ("MotorControlDevRef"=w955:T1)  [unwired: 9 in, 1 out]
          n299 = call <vilib>:"WPI_CANTalonSRX_SetReference.vi"("Reverse Closed-Loop Output"=TRUE, "Feedback Reference"=WPI_CANTalonSRX_APIFeedbackSelect."Count on Quad-A (Rising-Edge)", "CAN Talon SRX Ref"=w969) -> ("CAN Talon SRX Ref"=w970:T1)  [unwired: 7 in, 1 out]
          n300 = call <vilib>:"WPI_CANTalonSRX_SetReference.vi"("Reverse Closed-Loop Output"=TRUE, "Feedback Reference"=WPI_CANTalonSRX_APIFeedbackSelect."Count on Quad-A (Rising-Edge)", "CAN Talon SRX Ref"=w955) -> ("CAN Talon SRX Ref"=w956:T1)  [unwired: 7 in, 1 out]
          n301 = call-poly <vilib>:"NT Read Value.vi"("Name"="Top P") -> ("Numeric"=w961:dbl)  [unwired: 9 in, 1 out]
          n302 = call-poly <vilib>:"NT Read Value.vi"("Name"="Top I") -> ("Numeric"=w960:dbl)  [unwired: 9 in, 1 out]
          n303 = call-poly <vilib>:"NT Read Value.vi"("Name"="Bottom P") -> ("Numeric"=w947:dbl)  [unwired: 9 in, 1 out]
          n304 = call-poly <vilib>:"NT Read Value.vi"("Name"="Bottom I") -> ("Numeric"=w946:dbl)  [unwired: 9 in, 1 out]
          n305 = call-poly <vilib>:"NT Read Value.vi"("Name"="Top D") -> ("Numeric"=w959:dbl)  [unwired: 9 in, 1 out]
          n306 = call <vilib>:"WPI_CANTalonSRX_SetPID.vi"("CAN Talon SRX Ref"=w970, "P"=w961, "I"=w960, "D"=w959, "F"=0.0) -> ("CAN Talon SRX Ref"=w966:T1)  [unwired: 9 in, 1 out]
          n307 = call-poly <vilib>:"NT Read Value.vi"("Name"="Bottom D") -> ("Numeric"=w945:dbl)  [unwired: 9 in, 1 out]
          n308 = call <vilib>:"WPI_CANTalonSRX_SetPID.vi"("CAN Talon SRX Ref"=w956, "P"=w947, "I"=w946, "D"=w945, "F"=0.0) -> ("CAN Talon SRX Ref"=w952:T1)  [unwired: 9 in, 1 out]
          n309 = call-poly <vilib>:"NT Read Value.vi"("Name"="Bottom Speed") -> ("Numeric"=w929:dbl)  [unwired: 9 in, 1 out]
          n310 = call-poly <vilib>:"NT Read Value.vi"("Name"="Top Speed") -> ("Numeric"=w931:dbl)  [unwired: 9 in, 1 out]
          n311 = call <vilib>:"WPI_CANTalonSRX_ChangeMode.vi"("Output"=w931, "Control Mode"=WPI_CANTalonSRX_APIControlMode."Speed", "CAN Talon SRX Ref"=w966) -> ("CAN Talon SRX Ref"=w944:T1)  [unwired: 7 in, 1 out]
          n312 = call <vilib>:"WPI_CANTalonSRX_ChangeMode.vi"("Output"=w929, "Control Mode"=WPI_CANTalonSRX_APIControlMode."Speed", "CAN Talon SRX Ref"=w952) -> ("CAN Talon SRX Ref"=w943:T1)  [unwired: 7 in, 1 out]
        }
        frame #7 {
          n313 = call <vilib>:"WPI_MotorControlSetOutput.vi"("Output"=-0.8, "MotorControlDevRef"=w997) -> ("MotorControlDevRef"=w996:T1)  [unwired: 7 in, 2 out]
          n314 = call-poly <vilib>:"WPI_RobotDriveArcadeDrive.vi"("Y axis value"=0.0, "X axis value"=0.0, "RobotDriveDevRef"=w987) -> ("error out"=w991:errorcluster, "RobotDriveDevRef"=w986:T14)  [unwired: 6 in, 1 out]
          n315 = call <vilib>:"WPI_RobotDriveDelayAndUpdateSafety.vi"("error in (no error)"=w991, "Delay (s)"=2.0, "RobotDriveDevRef"=w986) -> ("RobotDriveDevRef 2"=w985:T14)  [unwired: 7 in, 1 out]
          n316 = call <vilib>:"WPI_CANTalonSRX_SetReference.vi"("Reverse Closed-Loop Output"=TRUE, "Feedback Reference"=WPI_CANTalonSRX_APIFeedbackSelect."Count on Quad-A (Rising-Edge)", "CAN Talon SRX Ref"=w993) -> ("CAN Talon SRX Ref"=w1020:T1)  [unwired: 7 in, 1 out]
          n317 = call <vilib>:"WPI_CANTalonSRX_SetReference.vi"("Reverse Closed-Loop Output"=TRUE, "Feedback Reference"=WPI_CANTalonSRX_APIFeedbackSelect."Count on Quad-A (Rising-Edge)", "CAN Talon SRX Ref"=w994) -> ("CAN Talon SRX Ref"=w1008:T1)  [unwired: 7 in, 1 out]
          n318 = call-poly <vilib>:"NT Read Value.vi"("Name"="Top P") -> ("Numeric"=w1013:dbl)  [unwired: 9 in, 1 out]
          n319 = call-poly <vilib>:"NT Read Value.vi"("Name"="Top I") -> ("Numeric"=w1012:dbl)  [unwired: 9 in, 1 out]
          n320 = call-poly <vilib>:"NT Read Value.vi"("Name"="Bottom P") -> ("Numeric"=w1001:dbl)  [unwired: 9 in, 1 out]
          n321 = call-poly <vilib>:"NT Read Value.vi"("Name"="Bottom I") -> ("Numeric"=w1000:dbl)  [unwired: 9 in, 1 out]
          n322 = call-poly <vilib>:"NT Read Value.vi"("Name"="Top D") -> ("Numeric"=w1011:dbl)  [unwired: 9 in, 1 out]
          n323 = call <vilib>:"WPI_CANTalonSRX_SetPID.vi"("CAN Talon SRX Ref"=w1020, "P"=w1013, "I"=w1012, "D"=w1011, "F"=0.0) -> ("CAN Talon SRX Ref"=w1018:T1)  [unwired: 9 in, 1 out]
          n324 = call-poly <vilib>:"NT Read Value.vi"("Name"="Bottom D") -> ("Numeric"=w999:dbl)  [unwired: 9 in, 1 out]
          n325 = call <vilib>:"WPI_CANTalonSRX_SetPID.vi"("CAN Talon SRX Ref"=w1008, "P"=w1001, "I"=w1000, "D"=w999, "F"=0.0) -> ("CAN Talon SRX Ref"=w1006:T1)  [unwired: 9 in, 1 out]
          n326 = call-poly <vilib>:"NT Read Value.vi"("Name"="Bottom Speed") -> ("Numeric"=w978:dbl)  [unwired: 9 in, 1 out]
          n327 = call-poly <vilib>:"NT Read Value.vi"("Name"="Top Speed") -> ("Numeric"=w980:dbl)  [unwired: 9 in, 1 out]
          n328 = call <vilib>:"WPI_CANTalonSRX_ChangeMode.vi"("Output"=w980, "Control Mode"=WPI_CANTalonSRX_APIControlMode."Speed", "CAN Talon SRX Ref"=w1018) -> ("CAN Talon SRX Ref"=w992:T1)  [unwired: 7 in, 1 out]
          n329 = call <vilib>:"WPI_CANTalonSRX_ChangeMode.vi"("Output"=w978, "Control Mode"=WPI_CANTalonSRX_APIControlMode."Speed", "CAN Talon SRX Ref"=w1006) -> ("CAN Talon SRX Ref"=w995:T1)  [unwired: 7 in, 1 out]
        }
        frame #8 {
          n330 = call-poly <vilib>:"WPI_RobotDriveArcadeDrive.vi"("Y axis value"=0.0, "X axis value"=0.0, "RobotDriveDevRef"=w1026) -> ()  [unwired: 6 in, 3 out]
          n331 = call <vilib>:"WPI_MotorControlSetOutput.vi"("Output"=0.0, "MotorControlDevRef"=w1024) -> ()  [unwired: 7 in, 3 out]
          n332 = call <vilib>:"WPI_MotorControlSetOutput.vi"("Output"=0.0, "MotorControlDevRef"=w1022) -> ()  [unwired: 7 in, 3 out]
          n333 = call <vilib>:"WPI_MotorControlSetOutput.vi"("Output"=0.0, "MotorControlDevRef"=w1030) -> ()  [unwired: 7 in, 3 out]
          n334 = call <vilib>:"WPI_CANTalonSRX_SetReference.vi"("Reverse Closed-Loop Output"=TRUE, "Feedback Reference"=WPI_CANTalonSRX_APIFeedbackSelect."Count on Quad-A (Rising-Edge)", "CAN Talon SRX Ref"=w1032) -> ("CAN Talon SRX Ref"=w1056:T1)  [unwired: 7 in, 1 out]
          n335 = call <vilib>:"WPI_CANTalonSRX_SetReference.vi"("Feedback Reference"=WPI_CANTalonSRX_APIFeedbackSelect."Count on Quad-A (Rising-Edge)", "CAN Talon SRX Ref"=w1029) -> ("CAN Talon SRX Ref"=w1044:T1)  [unwired: 8 in, 1 out]
          n336 = call-poly <vilib>:"NT Read Value.vi"("Name"="Top P") -> ("Numeric"=w1049:dbl)  [unwired: 9 in, 1 out]
          n337 = call-poly <vilib>:"NT Read Value.vi"("Name"="Top I") -> ("Numeric"=w1048:dbl)  [unwired: 9 in, 1 out]
          n338 = call-poly <vilib>:"NT Read Value.vi"("Name"="Bottom P") -> ("Numeric"=w1037:dbl)  [unwired: 9 in, 1 out]
          n339 = call-poly <vilib>:"NT Read Value.vi"("Name"="Bottom I") -> ("Numeric"=w1036:dbl)  [unwired: 9 in, 1 out]
          n340 = call-poly <vilib>:"NT Read Value.vi"("Name"="Top D") -> ("Numeric"=w1047:dbl)  [unwired: 9 in, 1 out]
          n341 = call <vilib>:"WPI_CANTalonSRX_SetPID.vi"("CAN Talon SRX Ref"=w1056, "P"=w1049, "I"=w1048, "D"=w1047, "F"=0.0) -> ("CAN Talon SRX Ref"=w1054:T1)  [unwired: 9 in, 1 out]
          n342 = call-poly <vilib>:"NT Read Value.vi"("Name"="Bottom D") -> ("Numeric"=w1035:dbl)  [unwired: 9 in, 1 out]
          n343 = call <vilib>:"WPI_CANTalonSRX_SetPID.vi"("CAN Talon SRX Ref"=w1044, "P"=w1037, "I"=w1036, "D"=w1035, "F"=0.0) -> ("CAN Talon SRX Ref"=w1042:T1)  [unwired: 9 in, 1 out]
          n344 = call <vilib>:"WPI_CANTalonSRX_ChangeMode.vi"("Output"=0.0, "Control Mode"=WPI_CANTalonSRX_APIControlMode."Percent VBus", "CAN Talon SRX Ref"=w1054) -> ()  [unwired: 7 in, 2 out]
          n345 = call <vilib>:"WPI_CANTalonSRX_ChangeMode.vi"("Output"=0.0, "Control Mode"=WPI_CANTalonSRX_APIControlMode."Percent VBus", "CAN Talon SRX Ref"=w1042) -> ()  [unwired: 7 in, 2 out]
        }
      }
    }
    frame 12 {
      n346 = flat-sequence {
        tunnel: w1058 -> [w1059]
        frame #0 {
          n347 = while {
            tunnel: w1059 -> [w1062]
            stop <- w1063 stop-if-true
            n348 = call-poly <vilib>:"NT Read Value.vi"("Name"="Angle Offset") -> ("Numeric"=w1074:dbl)  [unwired: 9 in, 1 out]
            n349 = call-poly <vilib>:"NT Read Value.vi"("Name"="Angle") -> ("Numeric"=w1075:dbl)  [unwired: 9 in, 1 out]
            n350 = call-poly <vilib>:"NT Read Value.vi"("Name"="Y Offset") -> ("Numeric"=w1064:dbl)  [unwired: 9 in, 1 out]
            n351 = call-poly <vilib>:"NT Read Value.vi"("Name"="Y") -> ("Numeric"=w1065:dbl)  [unwired: 9 in, 1 out]
            n352 = Greater?(x=w1075, y=w1074) -> (0:w1073:bool)
            n353 = Less?(x=w1075, y=w1074) -> (x < y?=w1072:bool)
            n354 = Greater Or Equal?(x=w1065, y=w1064) -> (x >= y?=w1063:bool)
            n355 = Select(t=-0.6, s=w1073, f=0.6) -> (s? t:f=w1060:dbl)
            n356 = Select(t=-0.6, s=w1072, f=0.6) -> (s? t:f=w1061:dbl)
            n357 = call <vilib>:"WPI_RobotDriveTankDrive.vi"("Right axis value"=w1060, "Left axis value"=w1061, "RobotDriveDevRef"=w1062) -> ()  [unwired: 6 in, 3 out]
          }
        }
      }
    }
    frame 11 {
      # "Vision Auto for 3 Position Drive Forward"
      n358 = flat-sequence {
        tunnel: w1125 -> [w1133]
        tunnel: w1124 -> [w1132]
        tunnel: w1123 -> [w1131]
        tunnel: [w1130] -> w1097
        tunnel: [w1129] -> w1095
        tunnel: w1118 -> [w1128]
        tunnel: [w1127] -> w1086
        tunnel: [w1126] -> w1082
        tunnel: w1097 -> [w1168]
        tunnel: [w1168] -> w1096
        tunnel: w1095 -> [w1167]
        tunnel: [w1165] -> w1094
        tunnel: [w1163] -> w1087
        tunnel: w1086 -> [w1163]
        tunnel: [w1162] -> w1083
        tunnel: w1082 -> [w1162]
        tunnel: w1096 -> [w1174]
        tunnel: [w1173] -> w1093
        tunnel: [w1172] -> w1092
        tunnel: w1094 -> [w1171]
        tunnel: [w1170] -> w1088
        tunnel: w1087 -> [w1170]
        tunnel: [w1169] -> w1084
        tunnel: w1083 -> [w1169]
        tunnel: w1093 -> [w1198]
        tunnel: [w1197] -> w1091
        tunnel: w1092 -> [w1200]
        tunnel: [w1199] -> w1090
        tunnel: [w1196] -> w1089
        tunnel: w1088 -> [w1196]
        tunnel: [w1195] -> w1085
        tunnel: w1084 -> [w1195]
        tunnel: w1091 -> [w1226]
        tunnel: [w1225] -> w1081
        tunnel: w1090 -> [w1228]
        tunnel: [w1227] -> w1079
        tunnel: w1089 -> [w1224]
        tunnel: w1085 -> [w1223]
        tunnel: w1081 -> [w1258]
        tunnel: [w1257] -> w1080
        tunnel: w1079 -> [w1256]
        tunnel: [w1255] -> w1078
        tunnel: w1080 -> [w1282]
        tunnel: w1078 -> [w1281]
        tunnel: [w1280] -> w1122
        tunnel: [w1279] -> w1121
        tunnel: w1122 -> [w1310]
        tunnel: w1121 -> [w1309]
        tunnel: [w1308] -> w1120
        tunnel: [w1307] -> w1119
        tunnel: w1120 -> [w1339]
        tunnel: w1119 -> [w1338]
        tunnel: [w1337] -> w1117
        tunnel: w1117 -> [w1372]
        tunnel: [w1371] -> w1116
        tunnel: w1114 -> [w1375]
        tunnel: w1113 -> [w1374]
        tunnel: w1112 -> [w1373]
        tunnel: [w1370] -> w1111
        tunnel: [w1369] -> w1110
        tunnel: w1116 -> [w1397]
        tunnel: w1115 -> [w1394]
        tunnel: w1111 -> [w1396]
        tunnel: w1110 -> [w1395]
        tunnel: [w1393] -> w1109
        tunnel: [w1392] -> w1108
        tunnel: [w1391] -> w1107
        tunnel: [w1390] -> w1106
        tunnel: [w1389] -> w1105
        tunnel: [w1388] -> w1104
        tunnel: w1109 -> [w1447]
        tunnel: w1108 -> [w1446]
        tunnel: w1107 -> [w1445]
        tunnel: w1106 -> [w1444]
        tunnel: w1105 -> [w1441]
        tunnel: w1104 -> [w1442]
        tunnel: [w1443] -> w1103
        tunnel: [w1442] -> w1102
        tunnel: [w1441] -> w1101
        tunnel: [w1440] -> w1100
        tunnel: [w1439] -> w1099
        tunnel: [w1438] -> w1098
        tunnel: w1103 -> [w1487]
        tunnel: w1102 -> [w1486]
        tunnel: w1101 -> [w1485]
        tunnel: w1100 -> [w1484]
        tunnel: w1099 -> [w1483]
        tunnel: w1098 -> [w1482]
        frame #0 {
          n359 = while {
            tunnel: w1133 -> [w1152]
            tunnel: w1132 -> [w1151]
            tunnel: w1131 -> [w1143]
            tunnel: [w1139] -> w1130
            tunnel: [w1138] -> w1129
            tunnel: w1128 -> [w1136]
            tunnel: [w1135] -> w1127
            tunnel: [w1134] -> w1126
            stop <- w1155 stop-if-true
            n360 = call <vilib>:"WPI_EncoderGet.vi"("EncoderDevRef"=w1151) -> ("Distance"=w1158:dbl, "EncoderDevRef"=w1135:T15)  [unwired: 5 in, 4 out]
            n361 = call <vilib>:"WPI_GyroGetAngle.vi"("GyroDevRef"=w1143) -> ("Angle"=w1149:dbl, "GyroDevRef"=w1139:T11)  [unwired: 6 in, 3 out]
            n362 = call <vilib>:"WPI_EncoderGet.vi"("EncoderDevRef"=w1152) -> ("Distance"=w1160:dbl, "EncoderDevRef"=w1134:T15)  [unwired: 5 in, 4 out]
            n363 = call-poly <vilib>:"NT Read Value.vi"("Name"="First Drive") -> ("Numeric"=w1157:dbl)  [unwired: 9 in, 1 out]
            n364 = Absolute Value(x=w1158) -> (abs(x)=w1154:dbl)
            n365 = Absolute Value(x=w1160) -> (abs(x)=w1153:dbl)
            n366 = Greater?(x=w1154, y=w1157) -> (0:w1156:bool)
            n367 = Greater?(x=w1153, y=w1157) -> (0:w1159:bool)
            n368 = Or(x=w1156, y=w1159) -> (x .or. y?=w1155:bool)
            n369 = Greater?(x=w1149, y=0.5) -> (0:w1145:bool)
            n370 = Less?(x=w1149, y=-0.5) -> (x < y?=w1147:bool)
            n371 = Select(t=-1.0, s=w1145, f=-0.9) -> (s? t:f=w1140:dbl)
            n372 = Select(t=-1.0, s=w1147, f=-0.9) -> (s? t:f=w1137:dbl)
            n373 = call <vilib>:"WPI_RobotDriveTankDrive.vi"("Right axis value"=w1140, "Left axis value"=w1137, "RobotDriveDevRef"=w1136) -> ("RobotDriveDevRef"=w1138:T14)  [unwired: 6 in, 2 out]
          }
        }
        frame #1 {
          n374 = call <vilib>:"WPI_RobotDriveTankDrive.vi"("RobotDriveDevRef"=w1167) -> ("RobotDriveDevRef"=w1166:T14)  [unwired: 8 in, 2 out]
          n375 = call <vilib>:"WPI_RobotDriveDelayAndUpdateSafety.vi"("Delay (s)"=0.5, "RobotDriveDevRef"=w1166) -> ("RobotDriveDevRef 2"=w1165:T14)  [unwired: 8 in, 1 out]
        }
        frame #2 {
          n376 = while {
            tunnel: w1174 -> [w1194]
            tunnel: [w1177] -> w1173
            tunnel: [w1176] -> w1172
            tunnel: w1171 -> [w1175]
            stop <- w1178 stop-if-true
            n377 = call <vilib>:"WPI_GyroGetAngle.vi"("GyroDevRef"=w1194) -> ("Angle"=w1181:dbl, "GyroDevRef"=w1176:T11)  [unwired: 6 in, 3 out]
            n378 = Greater?(x=w1181, y=1.0) -> (0:w1190:bool)
            n379 = Less?(x=w1181, y=-1.0) -> (x < y?=w1187:bool)
            n380 = Less?(x=w1181, y=1.0) -> (x < y?=w1179:bool)
            n381 = Greater?(x=w1181, y=-1.0) -> (0:w1180:bool)
            n382 = Select(t=-0.5, s=w1190, f=0.5) -> (s? t:f=w1185:dbl)
            n383 = Select(t=-0.5, s=w1187, f=0.5) -> (s? t:f=w1184:dbl)
            n384 = And(x=w1179, y=w1180) -> (x .and. y?=w1178:bool)
            n385 = call <vilib>:"WPI_RobotDriveTankDrive.vi"("Right axis value"=w1185, "Left axis value"=w1184, "RobotDriveDevRef"=w1175) -> ("RobotDriveDevRef"=w1177:T14)  [unwired: 6 in, 2 out]
          }
        }
        frame #3 {
          n386 = while {
            tunnel: w1200 -> [w1220]
            tunnel: [w1203] -> w1197
            tunnel: [w1201] -> w1199
            tunnel: w1198 -> [w1202]
            stop <- w1204 stop-if-true
            n387 = call <vilib>:"WPI_GyroGetAngle.vi"("GyroDevRef"=w1220) -> ("Angle"=w1207:dbl, "GyroDevRef"=w1201:T11)  [unwired: 6 in, 3 out]
            n388 = Greater?(x=w1207, y=91.0) -> (0:w1216:bool)
            n389 = Less?(x=w1207, y=89.0) -> (x < y?=w1213:bool)
            n390 = Less?(x=w1207, y=91.0) -> (x < y?=w1205:bool)
            n391 = Greater?(x=w1207, y=89.0) -> (0:w1206:bool)
            n392 = Select(t=-0.5, s=w1216, f=0.5) -> (s? t:f=w1211:dbl)
            n393 = Select(t=-0.5, s=w1213, f=0.5) -> (s? t:f=w1210:dbl)
            n394 = And(x=w1205, y=w1206) -> (x .and. y?=w1204:bool)
            n395 = call <vilib>:"WPI_RobotDriveTankDrive.vi"("Right axis value"=w1211, "Left axis value"=w1210, "RobotDriveDevRef"=w1202) -> ("RobotDriveDevRef"=w1203:T14)  [unwired: 6 in, 2 out]
          }
        }
        frame #4 {
          n396 = call <vilib>:"WPI_EncoderReset.vi"("EncoderDevRef"=w1223) -> ("EncoderDevRef"=w1221:T15)  [unwired: 9 in, 1 out]
          n397 = call <vilib>:"WPI_EncoderReset.vi"("EncoderDevRef"=w1224) -> ("EncoderDevRef"=w1222:T15)  [unwired: 9 in, 1 out]
          n398 = while {
            tunnel: w1222 -> [w1245]
            tunnel: w1228 -> [w1237]
            tunnel: [w1230] -> _
            tunnel: [w1233] -> w1225
            tunnel: w1226 -> [w1231]
            tunnel: [w1230] -> w1227
            tunnel: w1221 -> [w1229]
            stop <- w1248 stop-if-true
            n399 = call <vilib>:"WPI_EncoderGet.vi"("EncoderDevRef"=w1245) -> ("Distance"=w1251:dbl)  [unwired: 5 in, 5 out]
            n400 = call <vilib>:"WPI_GyroGetAngle.vi"("GyroDevRef"=w1237) -> ("Angle"=w1243:dbl, "GyroDevRef"=w1230:T11)  [unwired: 6 in, 3 out]
            n401 = call <vilib>:"WPI_EncoderGet.vi"("EncoderDevRef"=w1229) -> ("Distance"=w1253:dbl)  [unwired: 5 in, 5 out]
            n402 = call-poly <vilib>:"NT Read Value.vi"("Name"="Second Drive") -> ("Numeric"=w1250:dbl)  [unwired: 9 in, 1 out]
            n403 = Absolute Value(x=w1251) -> (abs(x)=w1247:dbl)
            n404 = Absolute Value(x=w1253) -> (abs(x)=w1246:dbl)
            n405 = Greater?(x=w1247, y=w1250) -> (0:w1249:bool)
            n406 = Greater?(x=w1246, y=w1250) -> (0:w1252:bool)
            n407 = Or(x=w1249, y=w1252) -> (x .or. y?=w1248:bool)
            n408 = Greater?(x=w1243, y=0.5) -> (0:w1239:bool)
            n409 = Less?(x=w1243, y=-0.5) -> (x < y?=w1241:bool)
            n410 = Select(t=-0.65, s=w1239, f=-0.6) -> (s? t:f=w1234:dbl)
            n411 = Select(t=-0.65, s=w1241, f=-0.6) -> (s? t:f=w1232:dbl)
            n412 = call <vilib>:"WPI_RobotDriveTankDrive.vi"("Right axis value"=w1234, "Left axis value"=w1232, "RobotDriveDevRef"=w1231) -> ("RobotDriveDevRef"=w1233:T14)  [unwired: 6 in, 2 out]
          }
        }
        frame #5 {
          n413 = while {
            tunnel: w1256 -> [w1278]
            tunnel: [w1259] -> _
            tunnel: [w1260] -> w1255
            tunnel: w1258 -> [w1261]
            tunnel: [w1259] -> w1257
            stop <- w1262 stop-if-true
            n414 = call <vilib>:"WPI_GyroGetAngle.vi"("GyroDevRef"=w1278) -> ("Angle"=w1265:dbl, "GyroDevRef"=w1260:T11)  [unwired: 6 in, 3 out]
            n415 = Greater?(x=w1265, y=1.0) -> (0:w1274:bool)
            n416 = Less?(x=w1265, y=-1.0) -> (x < y?=w1271:bool)
            n417 = Less?(x=w1265, y=1.0) -> (x < y?=w1263:bool)
            n418 = Greater?(x=w1265, y=-1.0) -> (0:w1264:bool)
            n419 = Select(t=-0.5, s=w1274, f=0.5) -> (s? t:f=w1269:dbl)
            n420 = Select(t=-0.5, s=w1271, f=0.5) -> (s? t:f=w1268:dbl)
            n421 = And(x=w1263, y=w1264) -> (x .and. y?=w1262:bool)
            n422 = call <vilib>:"WPI_RobotDriveTankDrive.vi"("Right axis value"=w1269, "Left axis value"=w1268, "RobotDriveDevRef"=w1261) -> ("RobotDriveDevRef"=w1259:T14)  [unwired: 6 in, 2 out]
          }
        }
        frame #6 {
          # "Drive Forward untill camera sees goal"
          n423 = while {
            tunnel: w1282 -> [w1294]
            tunnel: w1281 -> [w1295]
            tunnel: [w1293] -> w1280
            tunnel: [w1292] -> w1279
            stop <- w1283 stop-if-true
            n424 = call <vilib>:"WPI_GyroGetAngle.vi"("GyroDevRef"=w1295) -> ("Angle"=w1296:dbl, "GyroDevRef"=w1292:T11)  [unwired: 6 in, 3 out]
            n425 = Greater?(x=w1296, y=1.0) -> (0:w1303:bool)
            n426 = Less?(x=w1296, y=-1.0) -> (x < y?=w1300:bool)
            n427 = call-poly <vilib>:"NT Read Value.vi"("Name"="Y") -> ("Numeric"=w1290:dbl)  [unwired: 9 in, 1 out]
            n428 = Select(t=-0.5, s=w1303, f=-0.55) -> (s? t:f=w1298:dbl)
            n429 = call-poly <vilib>:"NT Read Value.vi"("Name"="X") -> ("Numeric"=w1288:dbl)  [unwired: 9 in, 1 out]
            n430 = Select(t=-0.5, s=w1300, f=-0.55) -> (s? t:f=w1297:dbl)
            n431 = Not Equal?(x=w1290, y=0.0) -> (x != y?=w1284:bool)
            n432 = Not Equal?(x=w1288, y=0.0) -> (x != y?=w1285:bool)
            n433 = And(x=w1285, y=w1284) -> (x .and. y?=w1283:bool)
            n434 = call <vilib>:"WPI_RobotDriveTankDrive.vi"("Right axis value"=w1298, "Left axis value"=w1297, "RobotDriveDevRef"=w1294) -> ("RobotDriveDevRef"=w1293:T14)  [unwired: 6 in, 2 out]
          }
        }
        frame #7 {
          n435 = while {
            tunnel: w1310 -> [w1325]
            tunnel: w1309 -> [w1326]
            tunnel: [w1312] -> w1308
            tunnel: [w1311] -> w1307
            stop <- w1313 stop-if-true
            n436 = call <vilib>:"WPI_GyroGetAngle.vi"("GyroDevRef"=w1326) -> ("GyroDevRef"=w1311:T11)  [unwired: 6 in, 4 out]
            n437 = call-poly <vilib>:"NT Read Value.vi"("Name"="Y") -> ("Numeric"=w1318:dbl)  [unwired: 9 in, 1 out]
            n438 = call-poly <vilib>:"NT Read Value.vi"("Name"="X") -> ("Numeric"=w1322:dbl)  [unwired: 9 in, 1 out]
            n439 = call-poly <vilib>:"NT Read Value.vi"("Name"="Y Offset") -> ("Numeric"=w1317:dbl)  [unwired: 9 in, 1 out]
            n440 = call-poly <vilib>:"NT Read Value.vi"("Name"="X Offset") -> ("Numeric"=w1321:dbl)  [unwired: 9 in, 1 out]
            n441 = Subtract(x=w1318, y=w1317) -> (x-y=w1314:dbl)
            n442 = Subtract(x=w1322, y=w1321) -> (x-y=w1320:dbl)
            n443 = Greater?(x=w1320, y=1.0) -> (0:w1333:bool)
            n444 = Less?(x=w1320, y=-1.0) -> (x < y?=w1330:bool)
            n445 = Select(t=-0.6, s=w1333, f=-0.65) -> (s? t:f=w1328:dbl)
            n446 = Select(t=-0.6, s=w1330, f=-0.65) -> (s? t:f=w1327:dbl)
            n447 = Greater?(x=w1314, y=0.0) -> (0:w1313:bool)
            n448 = call <vilib>:"WPI_RobotDriveTankDrive.vi"("Right axis value"=w1328, "Left axis value"=w1327, "RobotDriveDevRef"=w1325) -> ("RobotDriveDevRef"=w1312:T14)  [unwired: 6 in, 2 out]
          }
        }
        frame #8 {
          n449 = while {
            tunnel: w1339 -> [w1359]
            tunnel: w1338 -> [w1360]
            tunnel: [w1349] -> w1337
            stop <- w1350 stop-if-true
            n450 = call <vilib>:"WPI_GyroGetAngle.vi"("GyroDevRef"=w1360) -> ()  [unwired: 6 in, 5 out]
            n451 = call-poly <vilib>:"NT Read Value.vi"("Name"="Angle") -> ("Numeric"=w1353:dbl)  [unwired: 9 in, 1 out]
            n452 = call-poly <vilib>:"NT Read Value.vi"("Name"="Angle Offset") -> ("Numeric"=w1356:dbl)  [unwired: 9 in, 1 out]
            n453 = Subtract(x=w1353, y=w1356) -> (x-y=w1343:dbl)
            n454 = Greater?(x=w1343, y=1.0) -> (0:w1346:bool)
            n455 = Less?(x=w1343, y=180.0) -> (x < y?=w1347:bool)
            n456 = Less?(x=w1343, y=-1.0) -> (x < y?=w1341:bool)
            n457 = And(x=w1346, y=w1347) -> (x .and. y?=w1345:bool)
            n458 = Greater?(x=w1343, y=180.0) -> (0:w1342:bool)
            n459 = And(x=w1341, y=w1342) -> (x .and. y?=w1340:bool)
            n460 = Select(t=-0.5, s=w1345, f=0.5) -> (s? t:f=w1362:dbl)
            n461 = Select(t=-0.5, s=w1340, f=0.5) -> (s? t:f=w1361:dbl)
            n462 = Less?(x=w1343, y=1.0) -> (x < y?=w1351:bool)
            n463 = Greater?(x=w1343, y=-1.0) -> (0:w1352:bool)
            n464 = And(x=w1351, y=w1352) -> (x .and. y?=w1350:bool)
            n465 = call <vilib>:"WPI_RobotDriveTankDrive.vi"("Right axis value"=w1362, "Left axis value"=w1361, "RobotDriveDevRef"=w1359) -> ("RobotDriveDevRef"=w1349:T14)  [unwired: 6 in, 2 out]
          }
        }
        frame #9 {
          n466 = while {
            tunnel: w1375 -> [w1381]
            tunnel: [w1384] -> w1370
            tunnel: [w1383] -> w1369
            tunnel: w1373 -> [w1382]
            tunnel: w1374 -> [w1380]
            tunnel: w1372 -> [w1377]
            tunnel: [w1376] -> w1371
            stop <- w1385 stop-if-true
            n467 = call <vilib>:"WPI_MotorControlSetOutput.vi"("Output"=0.25, "MotorControlDevRef"=w1380) -> ("MotorControlDevRef"=w1384:T1)  [unwired: 7 in, 2 out]
            n468 = call <vilib>:"WPI_MotorControlSetOutput.vi"("Output"=-0.25, "MotorControlDevRef"=w1381) -> ("MotorControlDevRef"=w1383:T1)  [unwired: 7 in, 2 out]
            n469 = call <vilib>:"WPI_SwitchGetLimitValue.vi"("SwitchDevRef"=w1382) -> ("Switch Pressed"=w1385:bool)  [unwired: 8 in, 2 out]
            n470 = call <vilib>:"WPI_RobotDriveTankDrive.vi"("Right axis value"=0.0, "Left axis value"=0.0, "RobotDriveDevRef"=w1377) -> ("RobotDriveDevRef"=w1376:T14)  [unwired: 6 in, 2 out]
          }
        }
        frame #10 {
          n471 = call-poly <vilib>:"WPI_RobotDriveArcadeDrive.vi"("Y axis value"=0.0, "X axis value"=0.0, "RobotDriveDevRef"=w1397) -> ("error out"=w1436:errorcluster, "RobotDriveDevRef"=w1435:T14)  [unwired: 6 in, 1 out]
          n472 = call <vilib>:"WPI_RobotDriveDelayAndUpdateSafety.vi"("error in (no error)"=w1436, "Delay (s)"=3.0, "RobotDriveDevRef"=w1435) -> ("RobotDriveDevRef 2"=w1392:T14)  [unwired: 7 in, 1 out]
          n473 = call <vilib>:"WPI_MotorControlSetOutput.vi"("Output"=0.0, "MotorControlDevRef"=w1396) -> ("MotorControlDevRef"=w1388:T1)  [unwired: 7 in, 2 out]
          n474 = call <vilib>:"WPI_MotorControlSetOutput.vi"("Output"=0.0, "MotorControlDevRef"=w1395) -> ("MotorControlDevRef"=w1389:T1)  [unwired: 7 in, 2 out]
          n475 = call <vilib>:"WPI_MotorControlSetOutput.vi"("Output"=0.0, "MotorControlDevRef"=w1394) -> ("MotorControlDevRef"=w1391:T1)  [unwired: 7 in, 2 out]
          n476 = call <vilib>:"WPI_MotorControlRefNum Registry Get.vi"("refnum name"="Top Shooter") -> ("MotorControlDevRef"=w1430:T1)  [unwired: 9 in, 1 out]
          n477 = call <vilib>:"WPI_MotorControlRefNum Registry Get.vi"("refnum name"="Bottom Shooter") -> ("MotorControlDevRef"=w1416:T1)  [unwired: 9 in, 1 out]
          n478 = call <vilib>:"WPI_CANTalonSRX_SetReference.vi"("Reverse Closed-Loop Output"=TRUE, "Feedback Reference"=WPI_CANTalonSRX_APIFeedbackSelect."Count on Quad-A (Rising-Edge)", "CAN Talon SRX Ref"=w1430) -> ("CAN Talon SRX Ref"=w1431:T1)  [unwired: 7 in, 1 out]
          n479 = call <vilib>:"WPI_CANTalonSRX_SetReference.vi"("Reverse Closed-Loop Output"=TRUE, "Feedback Reference"=WPI_CANTalonSRX_APIFeedbackSelect."Count on Quad-A (Rising-Edge)", "CAN Talon SRX Ref"=w1416) -> ("CAN Talon SRX Ref"=w1417:T1)  [unwired: 7 in, 1 out]
          n480 = call-poly <vilib>:"NT Read Value.vi"("Name"="Top P") -> ("Numeric"=w1422:dbl)  [unwired: 9 in, 1 out]
          n481 = call-poly <vilib>:"NT Read Value.vi"("Name"="Top I") -> ("Numeric"=w1421:dbl)  [unwired: 9 in, 1 out]
          n482 = call-poly <vilib>:"NT Read Value.vi"("Name"="Bottom P") -> ("Numeric"=w1408:dbl)  [unwired: 9 in, 1 out]
          n483 = call-poly <vilib>:"NT Read Value.vi"("Name"="Bottom I") -> ("Numeric"=w1407:dbl)  [unwired: 9 in, 1 out]
          n484 = call-poly <vilib>:"NT Read Value.vi"("Name"="Top D") -> ("Numeric"=w1420:dbl)  [unwired: 9 in, 1 out]
          n485 = call <vilib>:"WPI_CANTalonSRX_SetPID.vi"("CAN Talon SRX Ref"=w1431, "P"=w1422, "I"=w1421, "D"=w1420, "F"=0.0) -> ("CAN Talon SRX Ref"=w1427:T1)  [unwired: 9 in, 1 out]
          n486 = call-poly <vilib>:"NT Read Value.vi"("Name"="Bottom D") -> ("Numeric"=w1406:dbl)  [unwired: 9 in, 1 out]
          n487 = call <vilib>:"WPI_CANTalonSRX_SetPID.vi"("CAN Talon SRX Ref"=w1417, "P"=w1408, "I"=w1407, "D"=w1406, "F"=0.0) -> ("CAN Talon SRX Ref"=w1413:T1)  [unwired: 9 in, 1 out]
          n488 = call-poly <vilib>:"NT Read Value.vi"("Name"="Bottom Speed") -> ("Numeric"=w1398:dbl)  [unwired: 9 in, 1 out]
          n489 = call-poly <vilib>:"NT Read Value.vi"("Name"="Top Speed") -> ("Numeric"=w1400:dbl)  [unwired: 9 in, 1 out]
          n490 = call <vilib>:"WPI_CANTalonSRX_ChangeMode.vi"("Output"=w1400, "Control Mode"=WPI_CANTalonSRX_APIControlMode."Speed", "CAN Talon SRX Ref"=w1427) -> ("CAN Talon SRX Ref"=w1393:T1)  [unwired: 7 in, 1 out]
          n491 = call <vilib>:"WPI_CANTalonSRX_ChangeMode.vi"("Output"=w1398, "Control Mode"=WPI_CANTalonSRX_APIControlMode."Speed", "CAN Talon SRX Ref"=w1413) -> ("CAN Talon SRX Ref"=w1390:T1)  [unwired: 7 in, 1 out]
        }
        frame #11 {
          n492 = call <vilib>:"WPI_MotorControlSetOutput.vi"("Output"=-0.8, "MotorControlDevRef"=w1445) -> ("MotorControlDevRef"=w1440:T1)  [unwired: 7 in, 2 out]
          n493 = call-poly <vilib>:"WPI_RobotDriveArcadeDrive.vi"("Y axis value"=0.0, "X axis value"=0.0, "RobotDriveDevRef"=w1446) -> ("error out"=w1457:errorcluster, "RobotDriveDevRef"=w1453:T14)  [unwired: 6 in, 1 out]
          n494 = call <vilib>:"WPI_RobotDriveDelayAndUpdateSafety.vi"("error in (no error)"=w1457, "Delay (s)"=2.0, "RobotDriveDevRef"=w1453) -> ("RobotDriveDevRef 2"=w1439:T14)  [unwired: 7 in, 1 out]
          n495 = call <vilib>:"WPI_CANTalonSRX_SetReference.vi"("Reverse Closed-Loop Output"=TRUE, "Feedback Reference"=WPI_CANTalonSRX_APIFeedbackSelect."Count on Quad-A (Rising-Edge)", "CAN Talon SRX Ref"=w1447) -> ("CAN Talon SRX Ref"=w1480:T1)  [unwired: 7 in, 1 out]
          n496 = call <vilib>:"WPI_CANTalonSRX_SetReference.vi"("Reverse Closed-Loop Output"=TRUE, "Feedback Reference"=WPI_CANTalonSRX_APIFeedbackSelect."Count on Quad-A (Rising-Edge)", "CAN Talon SRX Ref"=w1444) -> ("CAN Talon SRX Ref"=w1468:T1)  [unwired: 7 in, 1 out]
          n497 = call-poly <vilib>:"NT Read Value.vi"("Name"="Top P") -> ("Numeric"=w1473:dbl)  [unwired: 9 in, 1 out]
          n498 = call-poly <vilib>:"NT Read Value.vi"("Name"="Top I") -> ("Numeric"=w1472:dbl)  [unwired: 9 in, 1 out]
          n499 = call-poly <vilib>:"NT Read Value.vi"("Name"="Bottom P") -> ("Numeric"=w1461:dbl)  [unwired: 9 in, 1 out]
          n500 = call-poly <vilib>:"NT Read Value.vi"("Name"="Bottom I") -> ("Numeric"=w1460:dbl)  [unwired: 9 in, 1 out]
          n501 = call-poly <vilib>:"NT Read Value.vi"("Name"="Top D") -> ("Numeric"=w1471:dbl)  [unwired: 9 in, 1 out]
          n502 = call <vilib>:"WPI_CANTalonSRX_SetPID.vi"("CAN Talon SRX Ref"=w1480, "P"=w1473, "I"=w1472, "D"=w1471, "F"=0.0) -> ("CAN Talon SRX Ref"=w1478:T1)  [unwired: 9 in, 1 out]
          n503 = call-poly <vilib>:"NT Read Value.vi"("Name"="Bottom D") -> ("Numeric"=w1459:dbl)  [unwired: 9 in, 1 out]
          n504 = call <vilib>:"WPI_CANTalonSRX_SetPID.vi"("CAN Talon SRX Ref"=w1468, "P"=w1461, "I"=w1460, "D"=w1459, "F"=0.0) -> ("CAN Talon SRX Ref"=w1466:T1)  [unwired: 9 in, 1 out]
          n505 = call-poly <vilib>:"NT Read Value.vi"("Name"="Bottom Speed") -> ("Numeric"=w1448:dbl)  [unwired: 9 in, 1 out]
          n506 = call-poly <vilib>:"NT Read Value.vi"("Name"="Top Speed") -> ("Numeric"=w1450:dbl)  [unwired: 9 in, 1 out]
          n507 = call <vilib>:"WPI_CANTalonSRX_ChangeMode.vi"("Output"=w1450, "Control Mode"=WPI_CANTalonSRX_APIControlMode."Speed", "CAN Talon SRX Ref"=w1478) -> ("CAN Talon SRX Ref"=w1438:T1)  [unwired: 7 in, 1 out]
          n508 = call <vilib>:"WPI_CANTalonSRX_ChangeMode.vi"("Output"=w1448, "Control Mode"=WPI_CANTalonSRX_APIControlMode."Speed", "CAN Talon SRX Ref"=w1466) -> ("CAN Talon SRX Ref"=w1443:T1)  [unwired: 7 in, 1 out]
        }
        frame #12 {
          n509 = call-poly <vilib>:"WPI_RobotDriveArcadeDrive.vi"("Y axis value"=0.0, "X axis value"=0.0, "RobotDriveDevRef"=w1483) -> ()  [unwired: 6 in, 3 out]
          n510 = call <vilib>:"WPI_MotorControlSetOutput.vi"("Output"=0.0, "MotorControlDevRef"=w1486) -> ()  [unwired: 7 in, 3 out]
          n511 = call <vilib>:"WPI_MotorControlSetOutput.vi"("Output"=0.0, "MotorControlDevRef"=w1485) -> ()  [unwired: 7 in, 3 out]
          n512 = call <vilib>:"WPI_MotorControlSetOutput.vi"("Output"=0.0, "MotorControlDevRef"=w1484) -> ()  [unwired: 7 in, 3 out]
          n513 = call <vilib>:"WPI_CANTalonSRX_SetReference.vi"("Reverse Closed-Loop Output"=TRUE, "Feedback Reference"=WPI_CANTalonSRX_APIFeedbackSelect."Count on Quad-A (Rising-Edge)", "CAN Talon SRX Ref"=w1482) -> ("CAN Talon SRX Ref"=w1516:T1)  [unwired: 7 in, 1 out]
          n514 = call <vilib>:"WPI_CANTalonSRX_SetReference.vi"("Feedback Reference"=WPI_CANTalonSRX_APIFeedbackSelect."Count on Quad-A (Rising-Edge)", "CAN Talon SRX Ref"=w1487) -> ("CAN Talon SRX Ref"=w1504:T1)  [unwired: 8 in, 1 out]
          n515 = call-poly <vilib>:"NT Read Value.vi"("Name"="Top P") -> ("Numeric"=w1509:dbl)  [unwired: 9 in, 1 out]
          n516 = call-poly <vilib>:"NT Read Value.vi"("Name"="Top I") -> ("Numeric"=w1508:dbl)  [unwired: 9 in, 1 out]
          n517 = call-poly <vilib>:"NT Read Value.vi"("Name"="Bottom P") -> ("Numeric"=w1497:dbl)  [unwired: 9 in, 1 out]
          n518 = call-poly <vilib>:"NT Read Value.vi"("Name"="Bottom I") -> ("Numeric"=w1496:dbl)  [unwired: 9 in, 1 out]
          n519 = call-poly <vilib>:"NT Read Value.vi"("Name"="Top D") -> ("Numeric"=w1507:dbl)  [unwired: 9 in, 1 out]
          n520 = call <vilib>:"WPI_CANTalonSRX_SetPID.vi"("CAN Talon SRX Ref"=w1516, "P"=w1509, "I"=w1508, "D"=w1507, "F"=0.0) -> ("CAN Talon SRX Ref"=w1514:T1)  [unwired: 9 in, 1 out]
          n521 = call-poly <vilib>:"NT Read Value.vi"("Name"="Bottom D") -> ("Numeric"=w1495:dbl)  [unwired: 9 in, 1 out]
          n522 = call <vilib>:"WPI_CANTalonSRX_SetPID.vi"("CAN Talon SRX Ref"=w1504, "P"=w1497, "I"=w1496, "D"=w1495, "F"=0.0) -> ("CAN Talon SRX Ref"=w1502:T1)  [unwired: 9 in, 1 out]
          n523 = call <vilib>:"WPI_CANTalonSRX_ChangeMode.vi"("Output"=0.0, "Control Mode"=WPI_CANTalonSRX_APIControlMode."Percent VBus", "CAN Talon SRX Ref"=w1514) -> ()  [unwired: 7 in, 2 out]
          n524 = call <vilib>:"WPI_CANTalonSRX_ChangeMode.vi"("Output"=0.0, "Control Mode"=WPI_CANTalonSRX_APIControlMode."Percent VBus", "CAN Talon SRX Ref"=w1502) -> ()  [unwired: 7 in, 2 out]
        }
      }
    }
    frame 4 {
      # "STRAIGHT FORWARD AS FAST AS POSSIBLE"
      n525 = flat-sequence {
        tunnel: w1522 -> [w1529]
        tunnel: w1524 -> [_]
        tunnel: w1523 -> [_]
        tunnel: w1525 -> [_]
        tunnel: w1521 -> [_]
        tunnel: [w1528] -> w1520
        tunnel: w1519 -> [w1527]
        tunnel: w1518 -> [w1526]
        tunnel: w1520 -> [w1545]
        frame #0 {
          n526 = while {
            shift-right: [w1541] -> w1528
            shift-left: w1529 -> [w1543]
            tunnel: w1527 -> [w1531]
            tunnel: w1526 -> [w1530]
            stop <- w1534 stop-if-true
            n527 = call <vilib>:"WPI_RobotDriveTankDrive.vi"("Right axis value"=-1.0 ("Y axis value"), "Left axis value"=-1.0 ("X axis value"), "RobotDriveDevRef"=w1543) -> ("RobotDriveDevRef"=w1541:T14)  [unwired: 6 in, 2 out]
            n528 = call <vilib>:"WPI_EncoderGet.vi"("EncoderDevRef"=w1531) -> ("Distance"=w1537:dbl)  [unwired: 5 in, 5 out]
            n529 = call <vilib>:"WPI_EncoderGet.vi"("EncoderDevRef"=w1530) -> ("Distance"=w1539:dbl)  [unwired: 5 in, 5 out]
            n530 = call-poly <vilib>:"NT Read Value.vi"("Name"="First Drive") -> ("Numeric"=w1536:dbl)  [unwired: 9 in, 1 out]
            n531 = Absolute Value(x=w1537) -> (abs(x)=w1533:dbl)
            n532 = Absolute Value(x=w1539) -> (abs(x)=w1532:dbl)
            n533 = Greater?(x=w1533, y=w1536) -> (0:w1535:bool)
            n534 = Greater?(x=w1532, y=w1536) -> (0:w1538:bool)
            n535 = Or(x=w1535, y=w1538) -> (x .or. y?=w1534:bool)
          }
        }
        frame #1 {
          n536 = call-poly <vilib>:"WPI_RobotDriveArcadeDrive.vi"("Y axis value"=0.0, "X axis value"=0.0, "RobotDriveDevRef"=w1545) -> ()  [unwired: 6 in, 3 out]
        }
      }
    }
    frame 7 {
      # "SHIMMY OVER OBSTACLE"
      # "go over moat in auto"
      n537 = flat-sequence {
        tunnel: w1552 -> [w1560]
        tunnel: w1554 -> [_]
        tunnel: w1553 -> [_]
        tunnel: w1555 -> [_]
        tunnel: w1550 -> [_]
        tunnel: [w1559] -> w1551
        tunnel: w1550 -> [w1558]
        tunnel: w1549 -> [w1557]
        tunnel: w1548 -> [w1556]
        tunnel: w1551 -> [w1596]
        frame #0 {
          n538 = while {
            shift-right: [w1570] -> w1559
            shift-left: w1560 -> [w1580]
            tunnel: w1558 -> [w1563]
            tunnel: w1557 -> [w1562]
            tunnel: w1556 -> [w1561]
            stop <- w1573 stop-if-true
            n539 = call <vilib>:"WPI_GyroGetAngle.vi"("GyroDevRef"=w1563) -> ("Angle"=w1565:dbl)  [unwired: 6 in, 4 out]
            n540 = Absolute Value(x=w1565) -> (abs(x)=w1569:dbl)
            n541 = call <vilib>:"WPI_EncoderGet.vi"("EncoderDevRef"=w1562) -> ("Distance"=w1576:dbl)  [unwired: 5 in, 5 out]
            n542 = call <vilib>:"WPI_EncoderGet.vi"("EncoderDevRef"=w1561) -> ("Distance"=w1578:dbl)  [unwired: 5 in, 5 out]
            n543 = call-poly <vilib>:"NT Read Value.vi"("Name"="First Drive") -> ("Numeric"=w1575:dbl)  [unwired: 9 in, 1 out]
            n544 = Absolute Value(x=w1576) -> (abs(x)=w1572:dbl)
            n545 = Absolute Value(x=w1578) -> (abs(x)=w1571:dbl)
            n546 = Less?(x=w1569, y=5.0) -> (x < y?=w1567:bool)
            n547 = Greater?(x=w1572, y=w1575) -> (0:w1574:bool)
            n548 = Greater?(x=w1565, y=0.0) -> (0:w1564:bool)
            n549 = Greater?(x=w1571, y=w1575) -> (0:w1577:bool)
            n550 = Or(x=w1574, y=w1577) -> (x .or. y?=w1573:bool)
            n551 = case shown="False" w1567 {
              tunnel: w1580 -> [w1582 w1594]
              tunnel: [w1581 w1592] -> w1570
              tunnel: w1564 -> [w1583 _]
              frame False {
                n552 = case shown="True" w1583 {
                  tunnel: w1582 -> [w1584 w1590]
                  tunnel: [w1585 w1589] -> w1581
                  frame False {
                    n553 = call <vilib>:"WPI_RobotDriveTankDrive.vi"("Right axis value"=-0.8 ("Y axis value"), "Left axis value"=-1.0 ("X axis value"), "RobotDriveDevRef"=w1584) -> ("RobotDriveDevRef"=w1585:T14)  [unwired: 6 in, 2 out]
                  }
                  frame True {
                    n554 = call <vilib>:"WPI_RobotDriveTankDrive.vi"("Right axis value"=-1.0 ("Y axis value"), "Left axis value"=-0.8 ("X axis value"), "RobotDriveDevRef"=w1590) -> ("RobotDriveDevRef"=w1589:T14)  [unwired: 6 in, 2 out]
                  }
                }
              }
              frame True {
                n555 = call <vilib>:"WPI_RobotDriveTankDrive.vi"("Right axis value"=-1.0 ("Y axis value"), "Left axis value"=-1.0 ("X axis value"), "RobotDriveDevRef"=w1594) -> ("RobotDriveDevRef"=w1592:T14)  [unwired: 6 in, 2 out]
              }
            }
          }
        }
        frame #1 {
          n556 = call-poly <vilib>:"WPI_RobotDriveArcadeDrive.vi"("Y axis value"=0.0, "X axis value"=0.0, "RobotDriveDevRef"=w1596) -> ()  [unwired: 6 in, 3 out]
        }
      }
    }
    frame 0, Default {
      # "Drive under low bar using time and stop"
      n557 = flat-sequence {
        tunnel: [w1605] -> w1600
        tunnel: w1599 -> [w1604]
        tunnel: w1600 -> [w1608]
        frame #0 {
          n558 = call-poly <vilib>:"WPI_RobotDriveArcadeDrive.vi"("Y axis value"=-0.7, "X axis value"=0.1, "RobotDriveDevRef"=w1604) -> ("error out"=w1607:errorcluster, "RobotDriveDevRef"=w1606:T14)  [unwired: 6 in, 1 out]
          n559 = call <vilib>:"WPI_RobotDriveDelayAndUpdateSafety.vi"("error in (no error)"=w1607, "Delay (s)"=2.0, "RobotDriveDevRef"=w1606) -> ("RobotDriveDevRef 2"=w1605:T14)  [unwired: 7 in, 1 out]
        }
        frame #1 {
          n560 = call-poly <vilib>:"WPI_RobotDriveArcadeDrive.vi"("Y axis value"=0.0, "X axis value"=0.0, "RobotDriveDevRef"=w1608) -> ()  [unwired: 6 in, 3 out]
        }
      }
    }
    frame 6 {
      # "uses encoder values for low bar"
      n561 = flat-sequence {
        tunnel: w1614 -> [w1618]
        tunnel: [w1617] -> w1613
        tunnel: w1612 -> [w1616]
        tunnel: w1611 -> [w1615]
        tunnel: w1613 -> [w1634]
        frame #0 {
          n562 = while {
            shift-right: [w1630] -> w1617
            shift-left: w1618 -> [w1632]
            tunnel: [w1628] -> _
            tunnel: w1616 -> [w1620]
            tunnel: w1615 -> [w1619]
            stop <- w1623 stop-if-true
            w1625 = 130.0 ("y")
            n563 = call <vilib>:"WPI_EncoderGet.vi"("EncoderDevRef"=w1620) -> ("Distance"=w1629:dbl, "EncoderDevRef"=w1628:T15)  [unwired: 5 in, 4 out]
            n564 = call <vilib>:"WPI_EncoderGet.vi"("EncoderDevRef"=w1619) -> ("Distance"=w1626:dbl)  [unwired: 5 in, 5 out]
            n565 = Absolute Value(x=w1629) -> (abs(x)=w1622:dbl)
            n566 = call <vilib>:"WPI_RobotDriveTankDrive.vi"("Right axis value"=-0.65 ("Y axis value"), "Left axis value"=-0.65 ("X axis value"), "RobotDriveDevRef"=w1632) -> ("RobotDriveDevRef"=w1630:T14)  [unwired: 6 in, 2 out]
            n567 = Absolute Value(x=w1626) -> (abs(x)=w1621:dbl)
            n568 = Greater?(x=w1622, y=w1625) -> (0:w1627:bool)
            n569 = Greater?(x=w1621, y=w1625) -> (0:w1624:bool)
            n570 = Or(x=w1627, y=w1624) -> (x .or. y?=w1623:bool)
          }
        }
        frame #1 {
          n571 = call-poly <vilib>:"WPI_RobotDriveArcadeDrive.vi"("Y axis value"=0.0, "X axis value"=0.0, "RobotDriveDevRef"=w1634) -> ()  [unwired: 6 in, 3 out]
        }
      }
    }
  }
